vi "Main.vi"(11 "Module Admin":refnum<class "Delacor_lib_QMH_Module Admin.lvclass">) -> ()   [LabVIEW 2021, in "Panther Dashboard.lvlib"]
doc: "Panther Dashboard For DQMH®\n\nDeveloped and maintained by:\nPantherLAB\n\nMain Contributor- Developer:\n\n» Enrique Noé Arias\n\nBrainstorming & Code Reviews:\n\n» Matthias Baudot\n» Fabiola De La Cueva\n» Christopher Farmer\n» Cyril Gambini\n» Joerg Hampel\n» Olivier Jourdan\n» Cesar Muñoz\n» Darren Nattinger\n» Luis Orozco\n» Sam Taggart\n» Diego Torres"
uses:
  Panther Dashboard.lvlib
  <vilib>/Delacor/Delacor QMH/Libraries/Module Admin_class/Delacor_lib_QMH_Module Admin.lvclass
  Window Position--enum.ctl
  Module Data--cluster.ctl
  Maps List and refs--cluster.ctl
  <vilib>/National Instruments/Tree Map/Tree Map Data.ctl
  DQMH Modules Info--cluster.ctl
  Module type--enum.ctl
  Project References--cluster.ctl
  Selection Type--enum.ctl
  References Updated Argument--cluster.ctl
  Launch DQMH Scripting Tools Argument--cluster.ctl
  DQMH Tools Menu--enum.ctl
  <vilib>/Delacor/Delacor QMH/Libraries/Message Queue_class/Delacor_lib_QMH_Message Queue.lvclass/Delacor_lib_QMH_Message Queue.ctl
  Expand Results Argument--cluster.ctl
  Execute Default Event Request Argument--cluster.ctl
  Tree DQMH Selection Argument--cluster.ctl
  Scan DQMH Modules Argument--cluster.ctl
  Stop Argument--cluster.ctl
  Generate Project Documentation Argument--cluster.ctl
  Set App Theme Argument--cluster.ctl
  Show About Argument--cluster.ctl
  Update Module ID Argument--cluster.ctl
  Save Library Description Argument--cluster.ctl
  Save VI Description Argument--cluster.ctl
  Open Documentation Argument--cluster.ctl
  Save Project Documentation Argument--cluster.ctl
  Update Window Position Argument--cluster.ctl
  Public VIs names--enum.ctl
  <vilib>/Delacor/Delacor QMH/Libraries/Module Admin_class/Delacor_lib_QMH_Module Admin.lvclass/Delacor_lib_QMH_Module Admin.ctl
  <vilib>/Delacor/Delacor QMH/Libraries/Message Queue_class/Delacor_lib_QMH_Enqueue Message (Single).vi
  <vilib>/Delacor/Delacor QMH/Libraries/Module Admin_class/Delacor_lib_QMH_Get External Launch.vi
  Panther Dashboard--global.vi
  <vilib>/Platform/browser.llb/Open URL in Default Browser (path).vi
  <vilib>/Utility/error.llb/Error Cluster From Error Code.vi
  <vilib>/ErrorRing/Error Ring.xnode
  <vilib>/Delacor/Delacor QMH/Libraries/Message Queue_class/Delacor_lib_QMH_Message Queue.lvclass
  <vilib>/National Instruments/Tree Map/Tree Map.lvlib
  <vilib>/Delacor/Delacor QMH/Libraries/Scripting API/DQMH_Scripting API.lvlib
  ContextHelp/ContextHelp.lvlib
panel:
  out "error out":errorcluster
  in  "Context Help Panther":bool caption="Doc Editor"
  in  "Add Event":bool
  in  "Remove Event":bool caption="Remove"
  in  "Convert Event":bool caption="Convert"
  in  "Rename Event":bool caption="Rename"
  in  "Add Helper Loop to Module":bool
  in  "Add New Module":bool caption="Add"
  in  "Rename Module":bool caption="Rename"
  in  "Validate Module":bool caption="Validate"
  in  "Create Module Template":bool caption="Template"
  in  "Add Unit Test Module":bool caption="Unit Test"
  in  "Create RT Tester Module":bool caption="RT Tester"
  in  "Open Antidoc Output":bool caption="Open"
  in  "Generate Antidoc":bool caption="Antidoc"
  in  "About Panther":bool caption="About"
  in  "Theme Panther":bool caption="Theme"
  in  "Projects":string(combo)
  in  "Targets":string(combo)
  in  "Expand Results":bool
  in  "Include Dependencies":bool
  in  "Search All":bool caption="Scan All in Project"
  in  "Search":bool caption="Manual Scan Project"
  in  "Module ID":i32=-1 min=-1 max=1000 step=1 format="Module ID %d"
  in  "Modules Tree":string(tree) caption="Tree 2"
  out "antidoc":bool
  out "Panther Indicator":bool
  out "Process Indicator":bool
  out "Event Indicator":bool
  out "Status":string
  out "Progress":u16(slide) scale=-1.0..3.0
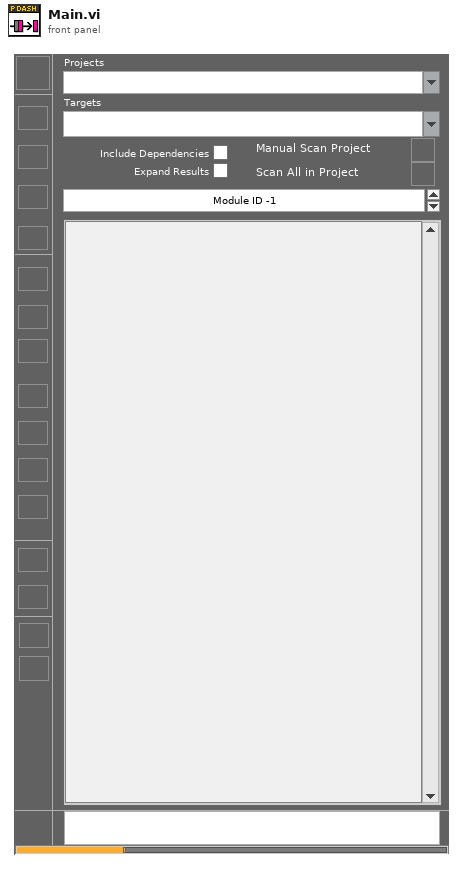
[diagram p1: front panel]
types:
  T1 = typedef "Panther Dashboard.lvlib/Window Position--enum.ctl" = enum16{"Right", "Left", "Max"}
  T2 = typedef "Panther Dashboard.lvlib/Broadcast Events--cluster.ctl" = cluster{"Module Did Init":refnum<user-event>, "Status Updated":refnum<user-event>, "Error Reported":refnum<user-event>, "Module Did Stop":refnum<user-event>, "Update Module Execution Status":refnum<user-event>, "References Updated":refnum<user-event>, "Projects Updated":refnum<user-event>, "Targets Updated":refnum<user-event>, "Progress updated":refnum<user-event>, "Scale Updated":refnum<user-event>, "Connector Pane Updated":refnum<user-event>, "Documentation Updated":refnum<user-event>, "Module Type Updated":refnum<user-event>, "Theme Updated":refnum<user-event>, "Project Description Updated":refnum<user-event>}
  T3 = typedef "Panther Dashboard.lvlib/Request Events--cluster.ctl" = cluster{"Stop Module":refnum<user-event>, "Show Panel":refnum<user-event>, "Hide Panel":refnum<user-event>, "Get Module Execution Status":refnum<user-event>, "Show Diagram":refnum<user-event>, "Scan DQMH Modules":refnum<user-event>, "Tree DQMH Selection":refnum<user-event>, "Open Module API Tester":refnum<user-event>, "Execute Default Event Request":refnum<user-event>, "Expand Results":refnum<user-event>, "Launch DQMH Scripting Tools":refnum<user-event>, "Generate Project Documentation":refnum<user-event>, "Set App Theme":refnum<user-event>, "Show About":refnum<user-event>, "Update Module ID":refnum<user-event>, "Save Library Description":refnum<user-event>, "Save VI Description":refnum<user-event>, "Open Documentation":refnum<user-event>, "Save Project Documentation":refnum<user-event>, "Register controls Mouse Enter":refnum<user-event>, "Update Window Position":refnum<user-event>}
  T4 = typedef "ContextHelp.lvlib/Broadcast Events--cluster.ctl" = cluster{"Module Did Init":refnum<user-event>, "Status Updated":refnum<user-event>, "Error Reported":refnum<user-event>, "Module Did Stop":refnum<user-event>, "Update Module Execution Status":refnum<user-event>}
  T5 = typedef "Panther Dashboard.lvlib/Selection Type--enum.ctl" = enum16{"Broadcast", "Request", "Module", "Public API"}
  T6 = typedef "Panther Dashboard.lvlib/Module Data--cluster.ctl" = cluster{"Maps":T7, "DQMH Scan Results":T9, "Current Selection":cluster{"VI Ref":refnum<vi>, "DQMH Lib Ref":refnum<vi>}, "Module type":T10, "Module ID":i32, "Theme":bool, "Broadcast?":bool}
  T7 = typedef "Panther Dashboard.lvlib/Maps List and refs--cluster.ctl" = cluster{"Tree Map":T8, "References Map":map{string, refnum<vi>}}
  T8 = typedef "Tree Map.lvlib/Tree Map Data.ctl" = map{string, cluster{"Child Paths Set":set{string}, "Name":string, "Data":string, "Attributes":map{string, string}}}
  T9 = typedef "Panther Dashboard.lvlib/DQMH Modules Info--cluster.ctl" = cluster{"All DQMH Modules Refs":refnum<vi>[], "All Modules Descriptions":string[], "All Modules type":T10[], "Project References":T11, "Dependencies":bool[]}
  T10 = typedef "Panther Dashboard.lvlib/Module type--enum.ctl" = enum16{"Module type: Singleton", "Module type: Cloneable"}
  T11 = typedef "Panther Dashboard.lvlib/Project References--cluster.ctl" = cluster{"Project Ref":refnum<vi>, "Project Name":string, "Target":refnum<vi>, "App Ref":refnum<vi>}
  T12 = typedef "Panther Dashboard.lvlib/References Updated Argument--cluster.ctl" = cluster{"Modules":refnum<vi>[], "Modules Types":T10[], "Application Instance":refnum<vi>, "Dependencies":bool[]}
  T13 = enum8{"Enabled", "Disabled", "Disabled and Grayed Out"}
  T14 = typedef "Panther Dashboard.lvlib/Launch DQMH Scripting Tools Argument--cluster.ctl" = cluster{"Scripting Tool":T15}
  T15 = typedef "Panther Dashboard.lvlib/DQMH Tools Menu--enum.ctl" = enum16{"Create New DQMH Event", "Remove DQMH Event", "Convert DQMH Event", "Rename DQMH Event", "Add New DQMH Module", "Create RT Tester", "Rename DQMH Module", "Validate DQMH Module", "Create DQMH Module Template", "New DQMH  Unit Test", "Add Helper Loop to DQMH Module"}
  T16 = typedef "Panther Dashboard.lvlib/Expand Results Argument--cluster.ctl" = cluster{"Expand?":bool}
  T17 = typedef "Panther Dashboard.lvlib/Execute Default Event Request Argument--cluster.ctl" = cluster{"Event Name":string}
  T18 = typedef "Panther Dashboard.lvlib/Tree DQMH Selection Argument--cluster.ctl" = cluster{"Tree DQMH Sel":string}
  T19 = typedef "Panther Dashboard.lvlib/Scan DQMH Modules Argument--cluster.ctl" = cluster{"Include Dependencies":bool, "Project":string, "Target":string, "All":bool}
  T20 = enum32{"invalid lock state", "Not Locked", "Locked (No Password)", "Password-protected"}
  T21 = typedef "Panther Dashboard.lvlib/Stop Argument--cluster.ctl" = cluster{"Origin":string, "Exit via Stop Module Req?":bool, "Wait for Module to stop?":bool}
  T22 = typedef "Panther Dashboard.lvlib/Generate Project Documentation Argument--cluster.ctl" = cluster{"Boolean":bool}
  T23 = typedef "Panther Dashboard.lvlib/Set App Theme Argument--cluster.ctl" = cluster{"Theme":bool}
  T24 = typedef "Panther Dashboard.lvlib/Show About Argument--cluster.ctl" = cluster{"Boolean":bool}
  T25 = typedef "Panther Dashboard.lvlib/Update Module ID Argument--cluster.ctl" = cluster{"New ID":i32}
  T26 = typedef "Panther Dashboard.lvlib/Save Library Description Argument--cluster.ctl" = cluster{"Library Description":string}
  T27 = typedef "Panther Dashboard.lvlib/Save VI Description Argument--cluster.ctl" = cluster{"VI Description":string}
  T28 = typedef "Panther Dashboard.lvlib/Open Documentation Argument--cluster.ctl" = cluster{"Boolean":bool}
  T29 = typedef "Panther Dashboard.lvlib/Save Project Documentation Argument--cluster.ctl" = cluster{"Project Description":string}
  T30 = typedef "Panther Dashboard.lvlib/Update Window Position Argument--cluster.ctl" = cluster{"Window Position":T1}
  T31 = typedef "Panther Dashboard.lvlib/Public VIs names--enum.ctl" = enum16{"Start Module.vi", "Synchronize Module Events.vi", "Obtain Broadcast Events for Registration.vi", "Null Broadcast Events--constant.vi", "Stop Module.vi"}
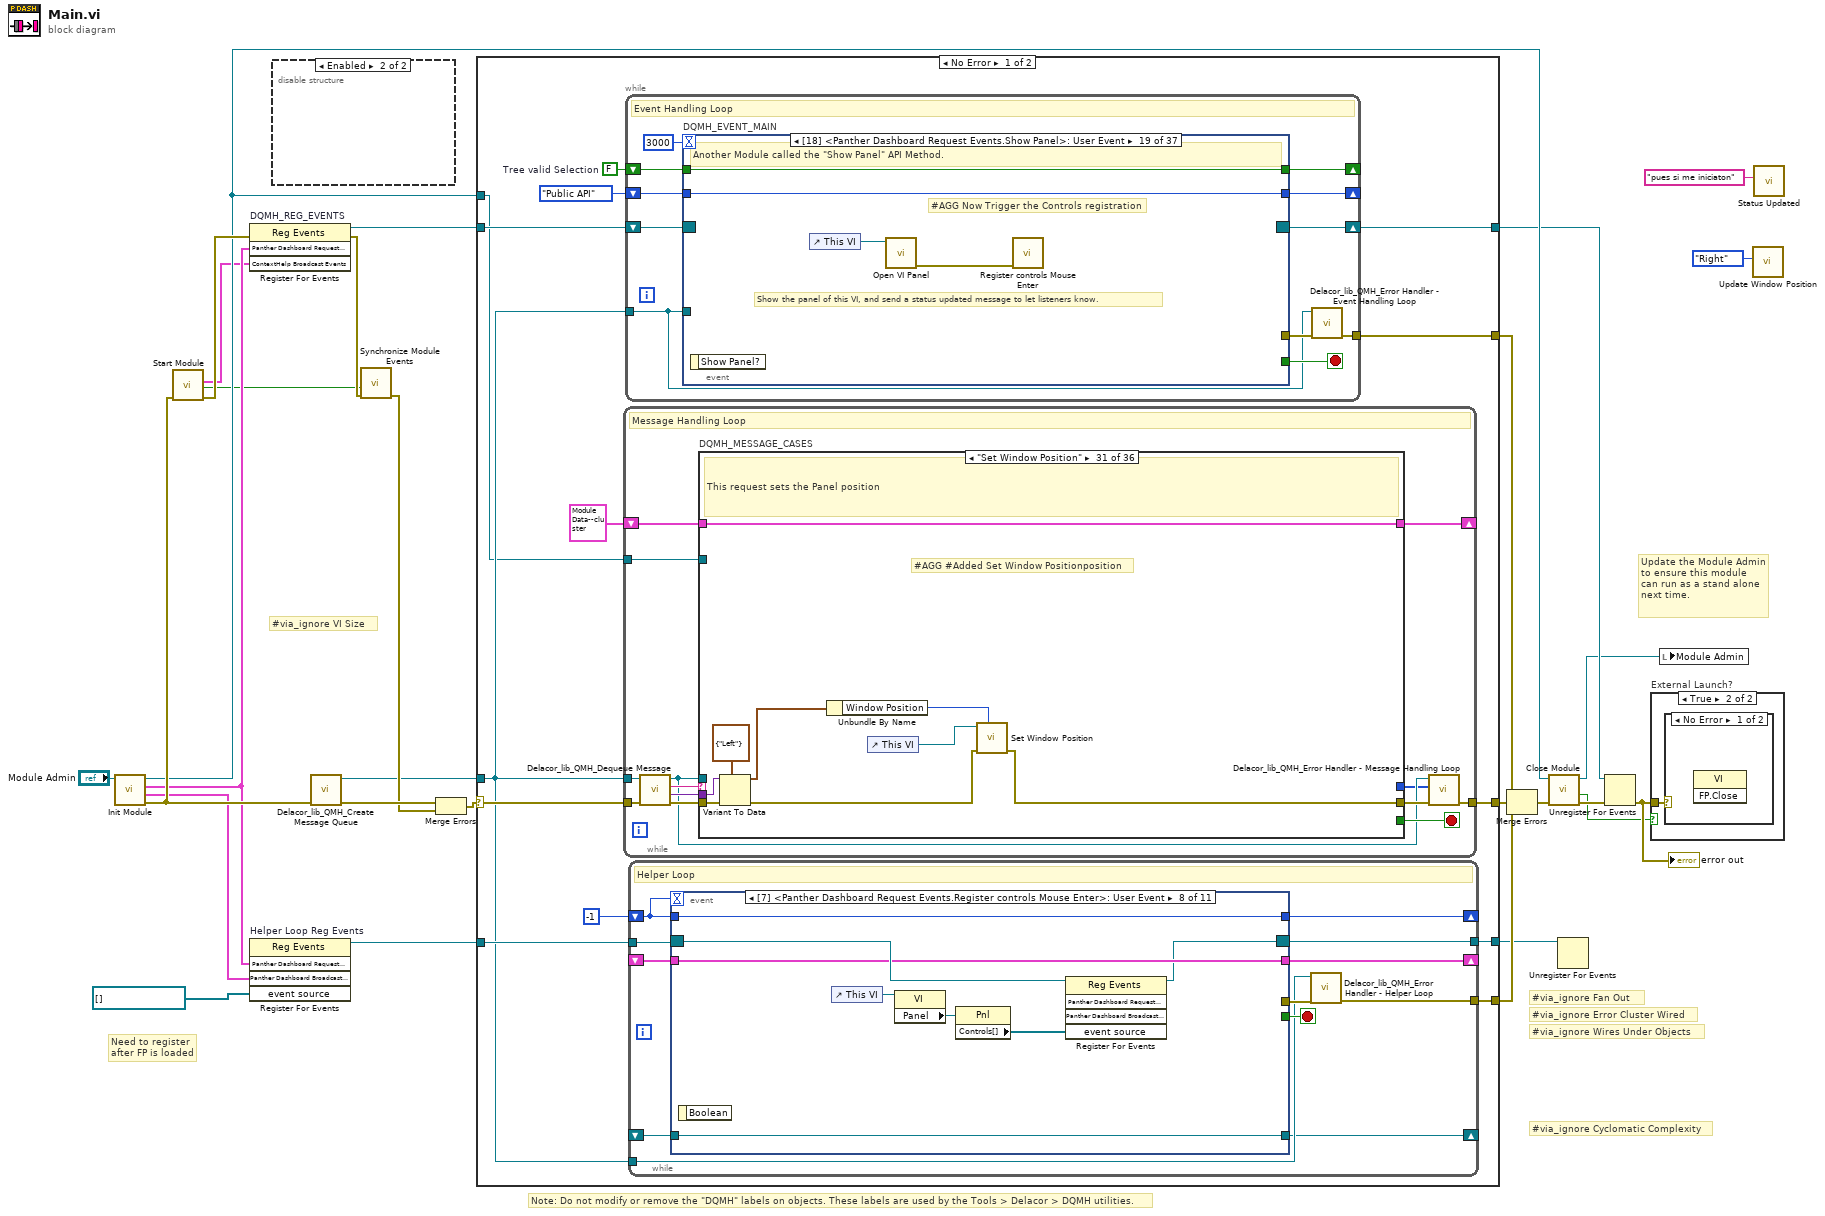
[diagram p0: block diagram]
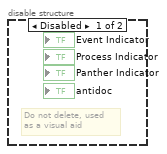
[diagram p2: hidden frame]
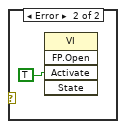
[diagram p4: hidden frame]
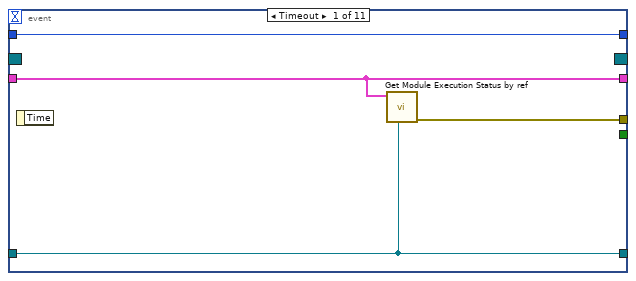
[diagram p5: hidden frame]
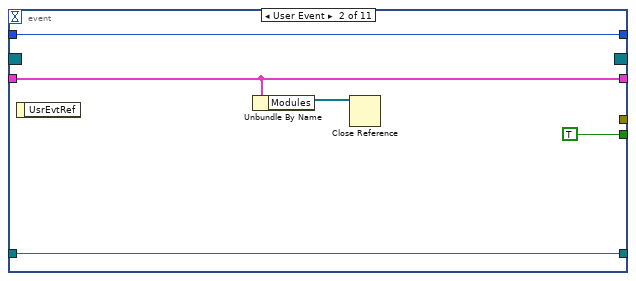
[diagram p6: hidden frame]
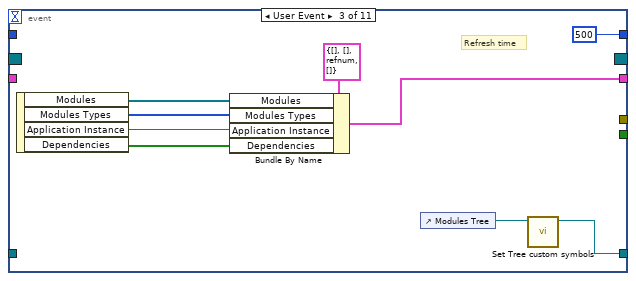
[diagram p7: hidden frame]
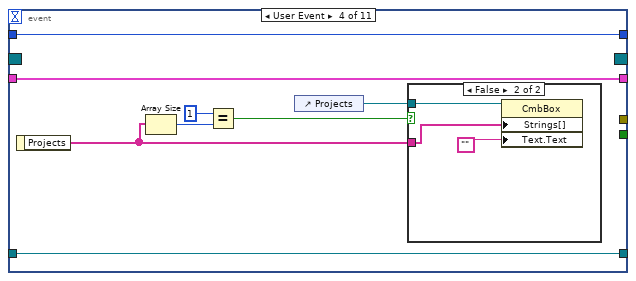
[diagram p8: hidden frame]
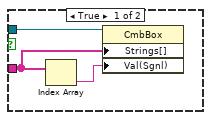
[diagram p9: hidden frame]
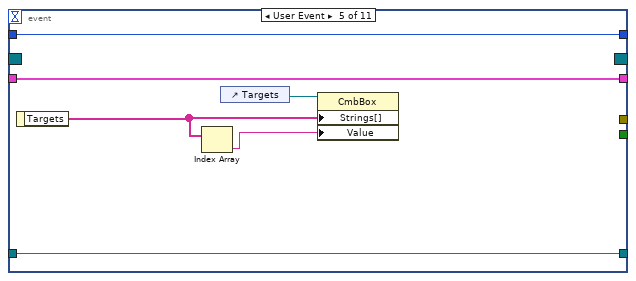
[diagram p10: hidden frame]
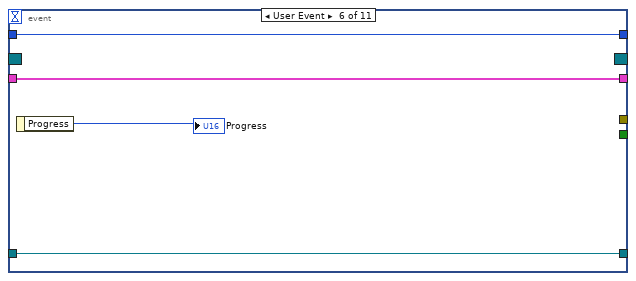
[diagram p11: hidden frame]
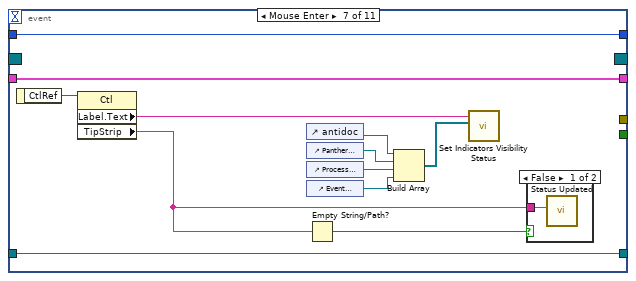
[diagram p12: hidden frame]
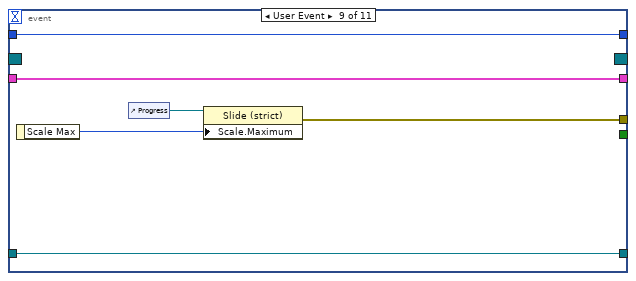
[diagram p14: hidden frame]
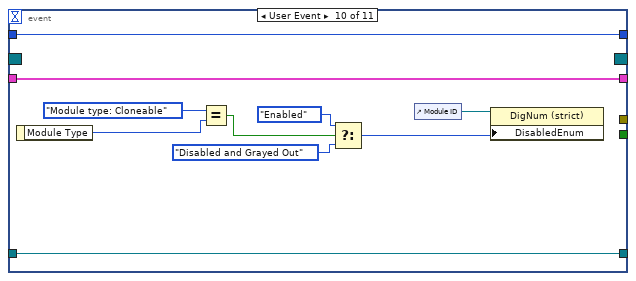
[diagram p15: hidden frame]
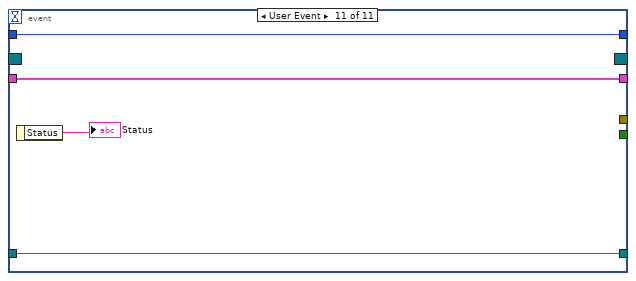
[diagram p16: hidden frame]
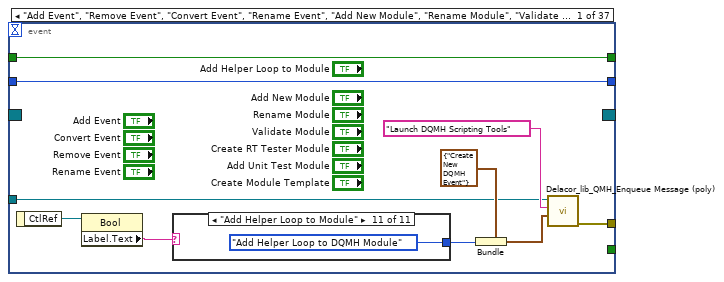
[diagram p17: hidden frame]
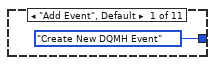
[diagram p18: hidden frame]
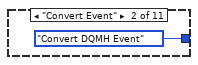
[diagram p19: hidden frame]
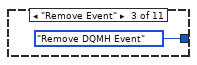
[diagram p20: hidden frame]
diagram:
  # "Need to register\nafter FP is loaded"
  # "#via_ignore VI Size"
  # "#via_ignore Fan Out"
  # "#via_ignore Cyclomatic Complexity"
  # "#via_ignore Wires Under Objects"
  # "#via_ignore Error Cluster Wired"
  # "Note: Do not modify or remove the \"DQMH\" labels on objects. These labels are used by the Tools > Delacor > DQMH utilities."
  # "Update the Module Admin to ensure this module can run as a stand alone next time."
  n1 = call "Init Module.vi"("Singleton Module Admin in"="Module Admin") -> ("error out"=w17:errorcluster, "Panther Dashboard Broadcast Events"=w6:T2, "Panther Dashboard Request Events"=w7:T3, "Singleton Module Admin out"=w16:refnum<class "Delacor_lib_QMH_Module Admin.lvclass">)  [unwired: 7 in]
  n2 = call "Start Module.vi"("error in"=w17) -> ("error out"=w19:errorcluster, "Wait for Event Sync?"=w5:bool, "ContextHelp Broadcast Events"=w4:T4)  [unwired: 7 in, 1 out]
  n3 = register-events "DQMH_REG_EVENTS"(error in=w19, w7, w4) -> (reference out=w14:refnum<event-registration>, error out=w20:errorcluster)  [unwired: 1 in]
  n4 = register-events "Helper Loop Reg Events"(w7, w6, refnum<vi>[] [] ("event source")) -> (reference out=w9:refnum<event-registration>)  [unwired: 2 in, 1 out]
  n5 = disable-structure shown="Enabled" {
    frame Disabled {
      # "Do not delete, used\nas a visual aid"
    }
    frame Enabled {
    }
  }
  n6 = call <vilib>:"Delacor_lib_QMH_Create Message Queue.vi"("error in"=w17) -> ("error out"=w23:errorcluster, "Message Queue"=w13:refnum<class "Delacor_lib_QMH_Message Queue.lvclass">)  [unwired: 9 in]
  n7 = call "Synchronize Module Events.vi"("error in"=w20, "Wait for Event Sync?"=w5) -> ("error out"=w18:errorcluster)  [unwired: 9 in]
  n8 = Merge Errors(w23, w18) -> (w22:errorcluster)
  n9 = case shown="No Error" w22 {
    selector: w22 -> [w40 w852]
    tunnel: [w42 w851] -> w28
    tunnel: [w38 w850] -> w15
    tunnel: w14 -> [w36 w850]
    tunnel: w13 -> [w32 w846]
    tunnel: [w41 _] -> w26
    tunnel: w16 -> [w29 w847]
    tunnel: w9 -> [w35 w845]
    tunnel: [w34 w845] -> w8
    tunnel: [w39 _] -> w21
    frame No Error {
      w31 = FALSE  # Tree valid Selection
      n10 = while {
        tunnel: w32 -> [w461]
        shift-right: [w465] -> _
        shift-left: T6 {"Maps"={"Tree Map"={}, "References Map"={}}, "DQMH Scan Results"={"All DQMH Modules Refs"=[], "All Modules Descriptions"=[], "All Modules type"=[], "Project References"={"Project Ref"=refnum, "Project Name"="", "Target"=refnum, "App Ref"=refnum}, "Dependencies"=[]}, "Current Selection"={"VI Ref"=refnum, "DQMH Lib Ref"=refnum}, "Module type"=enum."Module type: Singleton", "Module ID"=0, "Theme"=FALSE, "Broadcast?"=FALSE} ("Data Cluster") -> [w466]
        tunnel: w40 -> [w469]
        tunnel: [w467] -> w42
        tunnel: w29 -> [w459]
        stop <- w464 stop-if-true
        # "Message Handling Loop"
        n11 = call-dynamic "Delacor_lib_QMH_Dequeue Message.vi"("error in"=w469, "Message Queue in"=w461) -> ("error out"=w468:errorcluster, "Message Data"=w462:variant, "Message"=w463:string, "Message Queue out"=w460:refnum<class "Delacor_lib_QMH_Message Queue.lvclass">)  [unwired: 6 in]
        n12 = case "DQMH_MESSAGE_CASES" shown="\"Set Window Position\"" w463 {
          selector: w463 -> [_ w501 _ _ _ _ _ _ _ _ _ _ _ _ _ _ _ _ _ _ _ _ _ _ _ _ _ _ _ _ _ _ _ _ _ w831]
          tunnel: w460 -> [_ _ _ _ _ _ _ _ _ _ _ _ _ _ _ _ _ _ _ _ _ _ _ _ _ _ _ _ _ _ _ _ _ w800 w823 _]
          tunnel: w468 -> [w495 w506 w508 w521 w533 w540 w547 w554 w561 w576 w585 w590 w596 w610 w623 w645 w651 w657 w665 w672 w677 w690 w699 w710 w722 w730 w740 w756 w772 w783 w792 w795 w797 w807 w829 w833]
          tunnel: [w486 w504 w508 w510 w532 w539 w547 w554 w561 w575 w584 w591 w597 w608 w612 w646 w650 w658 w664 w671 w676 w688 w697 w707 w718 w729 w738 w754 w771 w781 w786 w794 w797 w803 w826 w834] -> w470
          tunnel: w466 -> [w489 w503 w507 w514 w531 w537 w546 w553 w560 w571 w583 w589 w595 w603 w622 w644 w649 w655 w663 w670 w675 w679 w693 w706 w717 w728 w732 w749 w761 w777 w791 w793 w796 w802 w815 w832]
          tunnel: [w493 w503 w507 w513 w530 w537 w546 w553 w560 w567 w583 w589 w595 w603 w622 w644 w649 w655 w661 w670 w675 w679 w693 w701 w717 w724 w731 w747 w761 w777 w791 w793 w796 w802 w815 w832] -> w465
          tunnel: [_ _ _ _ _ _ _ _ _ _ _ _ _ _ _ _ _ _ _ _ _ _ _ _ _ _ _ _ _ _ _ _ _ _ w822 _] -> w464
          tunnel: w462 -> [_ w502 _ w520 _ _ _ _ _ w574 _ _ _ w606 _ _ _ _ w662 w669 _ w687 w695 w705 w716 w727 w736 w752 w770 w780 w790 _ _ w801 w821 _]
          tunnel: w459 -> [w494 _ _ _ _ _ _ _ _ _ _ _ _ _ _ _ _ _ _ _ _ _ _ _ _ _ _ _ _ _ _ _ _ w799 w816 _]
          tunnel: [_ _ _ _ _ _ _ _ _ _ _ _ _ _ i32[] [5000, 1026, 43] ("specific error code to clear (0: all)") _ _ _ _ _ _ _ _ _ _ _ _ _ _ _ _ _ _ _ _ _] -> w458
          frame "Initialize" {
            # "Initialize - Any operation that needs to be done before the module can receive messages. Synchronize Caller Events.vi will inform Start Module.vi that the module has launched and is ready to receive messages. Module Did Init.vi will broadcast that the module initialized."
            n13 = call "Synchronize Caller Events.vi"("error in (no error)"=w495, "Singleton Module Admin in"=w494) -> ("error out"=w485:errorcluster)  [unwired: 8 in, 1 out]
            n14 = property on="Modules Tree" class="Tree (strict)"("Allow Item Drag"=TRUE ("Drag/Drop:Allow Dragging"), "SelColor"=u32 8355711) -> ()  [unwired: 2 in, 2 out]
            n15 = call "Module Name--constant.vi"() -> ("Module Name"=w483:string)  [unwired: 11 in]
            n16 = call "Module Did Init.vi"("error in (no error)"=w485, "Initialized?"=TRUE, "Origin"=w483) -> ("error out"=w482:errorcluster)  [unwired: 8 in]
            n17 = control-ref of="Projects"() -> (w478:refnum<vi>)
            n18 = control-ref of="Add Helper Loop to Module"() -> (w488:refnum<vi>)
            n19 = call "Scan For App Projects.vi"("error in"=w482, "Init?"=TRUE, "Projects Ref"=w478) -> ("error out"=w481:errorcluster)  [unwired: 8 in]
            n20 = call "Read Theme from Config.vi"("error in"=w481) -> ("error out"=w480:errorcluster, "Theme"=w475:bool)  [unwired: 9 in]
            n21 = local write "Theme Panther"(w475) -> ()
            n22 = call "Set App Theme.vi"("error in"=w480, "Theme"=w475) -> ("error out"=w472:errorcluster)  [unwired: 9 in]
            n23 = Build Array(w488) -> (w487:refnum<vi>[])
            n24 = call "Enable DQMH Version Caracteristics.vi"("Ctl Array"=w487) -> ()  [unwired: 11 in]
            n25 = control-ref of="This VI"() -> (w474:refnum<vi>)
            n26 = call "Update Window Position.vi"("error in"=w472, "Window Position"=Window_Position--enum."Right") -> ("error out"=w471:errorcluster)  [unwired: 9 in]
            n27 = flat-sequence {
              tunnel: [w498] -> w479
              tunnel: "Panther Dashboard for DQMH" ("format string") -> [w497]
              tunnel: w474 -> [w496]
              tunnel: w471 -> [_]
              frame #0 {
                n28 = call "Status Updated.vi"("Status"=w497) -> ()  [unwired: 10 in, 1 out]
                n29 = call "Set Panel Initial State.vi"("Title"=w497, "Main Vi Ref"=w496) -> ("error out"=w498:errorcluster)  [unwired: 9 in]
              }
            }
            n30 = Bundle By Name(cluster=w489, "Module ID"=-1) -> (w493:T6)
            n31 = Merge Errors(w479, w471) -> (w486:errorcluster)
          }
          frame "Refresh Targets" {
            # "When the User selects a Project triggers this task to scan all the targets available"
            n32 = Variant To Data(error in=w506, type=w501, Variant=w502) -> (data=w500:string, error out=w505:errorcluster)
            n33 = call "Get all Targets.vi"("error in"=w505, "Project Selection"=w500) -> ("error out"=w504:errorcluster, "Targets"=w499:string[])  [unwired: 8 in]
            n34 = call "Targets Updated.vi"("Targets"=w499) -> ()  [unwired: 10 in, 1 out]
          }
          frame "---Module Specific---" {
            # "Separator -- The following cases handle messages specific to this Module."
          }
          frame "Scan DQMH Modules" {
            # "Scan DQMH Modules in the project and fill 2 maps one with the Vi References and the another one with the list of DQMH modules on the project"
            n35 = Variant To Data(error in=w521, type=T19 {"Include Dependencies"=FALSE, "Project"="", "Target"="", "All"=FALSE} ("Scan DQMH Modules Argument"), Variant=w520) -> (data=w518:T19, error out=w511:errorcluster)
            n36 = Unbundle By Name(w518) -> ("Project"=w515:string, "Target"=w516:string, "Include Dependencies"=w517:bool, "All"=w509:bool)
            n37 = call <vilib>:"Set Busy.vi"("error in (no error)"=w511) -> ()  [unwired: 9 in, 2 out]
            n38 = control-ref of="Modules Tree"() -> (w512:refnum<vi>)
            n39 = call "Scan DQMH Modules and create Maps.vi"("All"=w509, "TreeControl in"=w512, "Data Cluster In"=w514, "error in"=w511, "Include Dependencies"=w517, "Target Selection"=w516, "Project"=w515) -> ("error out"=w510:errorcluster, "Data Cluster Out"=w513:T6)  [unwired: 3 in]
            n40 = call <vilib>:"Unset Busy.vi"("error in (no error)"=w510) -> ()  [unwired: 10 in, 1 out]
            n41 = local write "Include Dependencies"(w517) -> ()
          }
          frame "Refresh Module" {
            # "User right click a module and selected Refresh module"
            n42 = Unbundle By Name(w531) -> ("DQMH Scan Results.Project References.App Ref"=w524:refnum<vi>, "Current Selection.DQMH Lib Ref"=w525:refnum<vi>, "Maps.Tree Map"=w527:T8, "Maps.References Map"=w526:map{string, refnum<vi>})
            n43 = local read "Expand Results"() -> (w523:bool)
            n44 = control-ref of="Modules Tree"() -> (w522:refnum<vi>)
            n45 = call "Refresh Current DQMH Module.vi"("TreeControl in"=w522, "App Ref"=w524, "Expand Results"=w523, "DQMH Lib Ref"=w525, "error in"=w533, "References Map"=w526, "Tree Map In"=w527) -> ("error out"=w532:errorcluster, "map ref out"=w529:map{string, refnum<vi>}, "Tree Map out"=w528:T8)  [unwired: 2 in]
            n46 = Bundle By Name(cluster=w531, "Maps.Tree Map"=w528, "Maps.References Map"=w529) -> (w530:T6)
          }
          frame "Drag VI" {
            # "This is the functionality alowing drag and drop the current selection to your code, you can build code using panther Dashboard."
            n47 = Unbundle By Name(w537) -> ("DQMH Scan Results.Project References.App Ref"=w536:refnum<vi>, "DQMH Scan Results.Project References.Target"=w535:refnum<vi>, "Current Selection.VI Ref"=w534:refnum<vi>)
            n48 = call "Drop Event into subVI.vi"("Current Selection.VI Ref"=w534, "Target"=w535, "App Ref"=w536) -> ("error out"=w538:errorcluster)  [unwired: 8 in]
            n49 = Merge Errors(w538, w540) -> (w539:errorcluster)
          }
          frame "Where is this module being Launched?" {
            # "Find all the VIS calling the Start Module.vi of the selected module library"
            n50 = Unbundle By Name(w546) -> ("Theme"=w545:bool, "DQMH Scan Results.Project References.App Ref"=w544:refnum<vi>, "DQMH Scan Results.Project References.Target"=w543:refnum<vi>, "Current Selection.DQMH Lib Ref"=w542:refnum<vi>)
            n51 = call "Find some Public API VI.vi"("Theme"=w545, "Framework VI to Find"=Public_VIs_names--enum."Start Module.vi", "Library in"=w542, "Target"=w543, "App Ref"=w544) -> ()  [unwired: 7 in]
          }
          frame "Find Code registered to this module's broadcasts" {
            # "Find all the VIS calling the Obtain broadcast events for registration of the selected module library"
            n52 = Unbundle By Name(w553) -> ("Theme"=w551:bool, "DQMH Scan Results.Project References.App Ref"=w550:refnum<vi>, "DQMH Scan Results.Project References.Target"=w549:refnum<vi>, "Current Selection.DQMH Lib Ref"=w548:refnum<vi>)
            n53 = call "Find some Public API VI.vi"("Theme"=w551, "Framework VI to Find"=Public_VIs_names--enum."Obtain Broadcast Events for Registration.vi", "Library in"=w548, "Target"=w549, "App Ref"=w550) -> ()  [unwired: 7 in]
          }
          frame "Where is this module being Stopped?" {
            # "Find all the VIS calling the Obtain broadcast events for registration of the selected module library"
            n54 = Unbundle By Name(w560) -> ("Theme"=w558:bool, "DQMH Scan Results.Project References.App Ref"=w557:refnum<vi>, "DQMH Scan Results.Project References.Target"=w556:refnum<vi>, "Current Selection.DQMH Lib Ref"=w555:refnum<vi>)
            n55 = call "Find some Public API VI.vi"("Theme"=w558, "Framework VI to Find"=Public_VIs_names--enum."Stop Module.vi", "Library in"=w555, "Target"=w556, "App Ref"=w557) -> ()  [unwired: 7 in]
          }
          frame "Tree DQMH Selection" {
            # "There is a new selection of the DQMH Tree list, need to search and update indicators acordanly."
            n56 = Unbundle By Name(w571) -> ("Maps.Tree Map"=w570:T8, "Maps.References Map"=w569:map{string, refnum<vi>}, "DQMH Scan Results"=w568:T9)
            n57 = Variant To Data(error in=w576, type=T18 {"Tree DQMH Sel"=""} ("Tree DQMH Selection Argument"), Variant=w574) -> (data=w572:T18, error out=w575:errorcluster)
            n58 = Unbundle By Name(w572) -> ("Tree DQMH Sel"=w565:string)
            n59 = call "Get List Information.vi"("List Selection"=w565, "DQMH Scan Info"=w568, "References Map"=w569, "Tree Map"=w570) -> ("Broadcast?"=w564:bool, "Vi out"=w563:refnum<vi>, "Module type"=w562:T10, "DQMH Lib"=w566:refnum<vi>)  [unwired: 4 in]
            n60 = Bundle By Name(cluster=w571, "Current Selection.DQMH Lib Ref"=w566, "Module type"=w562, "Current Selection.VI Ref"=w563, "Broadcast?"=w564) -> (w567:T6)
          }
          frame "Open Module API Tester" {
            # "If nothing selected use the first DQMH module"
            # "Open the API Tester from the current DQMH Module Selected"
            n61 = Unbundle By Name(w583) -> ("DQMH Scan Results.Project References.App Ref"=w582:refnum<vi>, "DQMH Scan Results.All DQMH Modules Refs"=w581:refnum<vi>[], "Current Selection.DQMH Lib Ref"=w577:refnum<vi>)
            n62 = Index Array(array=w581) -> (element=w579:refnum<vi>)  [unwired: 1 in]
            n63 = Not A Number/Path/Refnum?(number/path/refnum=w577) -> (NaN/Path/Refnum?=w580:bool)
            n64 = Select(t=w579, s=w580, f=w577) -> (s? t:f=w578:refnum<vi>)
            n65 = call "Open API Tester.vi"("error in"=w585, "DQMH Library Ref"=w578, "Application Instance"=w582) -> ("error out"=w584:errorcluster)  [unwired: 8 in]
          }
          frame "Find Module in project" {
            # "Find the selected module in project explorer"
            n66 = Unbundle By Name(w589) -> ("Current Selection.DQMH Lib Ref"=w588:refnum<vi>, "DQMH Scan Results.Project References.Project Ref"=w587:refnum<vi>, "DQMH Scan Results.All DQMH Modules Refs"=w586:refnum<vi>[])
            n67 = call "Find Library in Project.vi"("error in (no error)"=w590, "DQMH Modules Refs"=w586, "Project Ref"=w587, "DQMH Lib Ref"=w588) -> ("error out"=w591:errorcluster)  [unwired: 7 in]
          }
          frame "Locate Event on Main" {
            # "Find the selected event vi on the owing DQMH Module, if it is a reques we highlight its frame, if it is a broadcast we highlight where the broadcast is being triggered"
            n68 = Unbundle By Name(w595) -> ("DQMH Scan Results.Project References.App Ref"=w593:refnum<vi>, "Current Selection.VI Ref"=w594:refnum<vi>, "Broadcast?"=w592:bool)
            n69 = call "Find Event Frame.vi"("error in"=w596, "Broadcast?"=w592, "VI in"=w594, "Application Instance"=w593) -> ("error out"=w597:errorcluster)  [unwired: 7 in]
          }
          frame "Execute Default Event Request" {
            # "Execute Default Event"
            n70 = Variant To Data(error in=w610, type=T17 {"Event Name"=""} ("Execute Default Event Request Argument"), Variant=w606) -> (data=w604:T17, error out=w609:errorcluster)
            n71 = Unbundle By Name(w603) -> ("DQMH Scan Results.Project References.App Ref"=w602:refnum<vi>, "Current Selection.DQMH Lib Ref"=w601:refnum<vi>, "Module ID"=w599:i32, "Module type"=w598:T10)
            n72 = Unbundle By Name(w604) -> ("Event Name"=w600:string)
            n73 = call "Execute Default event.vi"("Module type"=w598, "Module ID"=w599, "Event"=w600, "DQMH Library Ref"=w601, "application Instance"=w602) -> ("error out"=w607:errorcluster)  [unwired: 6 in]
            n74 = Merge Errors(w609, w607) -> (w608:errorcluster)
          }
          frame "Search for Event Callers / listeners" {
            # "1026-Invalid Ref\n43- Operation\n canceled by user\n5000- something\nrandom happening\non DQMH Scripting\nAPI"
            # "Search for this event callers"
            n75 = Unbundle By Name(w622) -> ("DQMH Scan Results.Project References.Project Ref"=w616:refnum<vi>, "Current Selection.VI Ref"=w621:refnum<vi>, "Theme"=w613:bool, "Broadcast?"=w614:bool)
            n76 = Select(t="Searching code registered to broadcast selection" ("Status"), s=w614, f="Searching for Event Callers" ("Status")) -> (s? t:f=w617:string)
            n77 = call "Status Updated.vi"("error in (no error)"=w623, "Status"=w617) -> ("error out"=w611:errorcluster)  [unwired: 9 in]
            n78 = case shown="True" w614 {
              tunnel: w611 -> [w628 w635]
              tunnel: [w627 w634] -> w612
              tunnel: w621 -> [w626 w631]
              tunnel: [w625 w633] -> w620
              tunnel: w616 -> [w624 w632]
              frame False {
                # "Requests"
                n79 = call <vilib>:"Get Callers of Request VI in Project.vi"("error in"=w628, "Request VI"=w626, "Project"=w624) -> ("error out"=w627:errorcluster, "Request VI Callers"=w625:refnum<vi>[])  [unwired: 7 in]
              }
              frame True {
                # "Broadcast"
                n80 = Two Button Dialog(message="This is an exhaustive task that can take up to minutes, do you wish to continue?") -> (T button?=w630:bool)  [unwired: 2 in]
                n81 = case shown="True" w630 {
                  tunnel: w635 -> [w636 w641]
                  tunnel: [w636 w640] -> w634
                  tunnel: [_ w639] -> w633
                  tunnel: w632 -> [_ w638]
                  tunnel: w631 -> [_ w637]
                  frame False {
                  }
                  frame True {
                    n82 = call <vilib>:"Get VIs Registered for Broadcast in Project.vi"("error in"=w641, "Broadcast VI"=w637, "Project"=w638) -> ("error out"=w640:errorcluster, "VIs Registered for Broadcast"=w639:refnum<vi>[])  [unwired: 7 in]
                  }
                }
              }
            }
            n83 = call <vilib>:"Set Busy.vi"("error in (no error)"=w611) -> ()  [unwired: 9 in, 2 out]
            n84 = call <vilib>:"Unset Busy.vi"("error in (no error)"=w612) -> ()  [unwired: 10 in, 1 out]
            n85 = call "Start Call to results window.vi"("Find Broadcast?"=w614, "Request VI Callers"=w620, "Event"=w621, "Theme"=w613) -> ()  [unwired: 8 in]
          }
          frame "Open VI on Disk" {
            # "Open current event selection on the file system"
            n86 = Unbundle By Name(w644) -> ("Current Selection.VI Ref"=w643:refnum<vi>)
            n87 = property class="VI"(reference=w643) -> ("Path"=w642:path)  [unwired: 1 in, 2 out]
            n88 = call "Open File on Disk.vi"("error in"=w645, "file or directory path"=w642) -> ("error out"=w646:errorcluster)  [unwired: 9 in]
          }
          frame "Open File Library on Disk" {
            # "Open current Module Library selection on the file system"
            n89 = Unbundle By Name(w649) -> ("Current Selection.DQMH Lib Ref"=w648:refnum<vi>)
            n90 = property class="Library"(reference=w648) -> ("Path"=w647:path)  [unwired: 1 in, 2 out]
            n91 = call "Open File on Disk.vi"("error in"=w651, "file or directory path"=w647) -> ("error out"=w650:errorcluster)  [unwired: 9 in]
          }
          frame "Open Event Arguments" {
            # "Open The event selected DQMH Arguments, also open the Event BD to do edits on it"
            n92 = Unbundle By Name(w655) -> ("Current Selection.VI Ref"=w654:refnum<vi>)
            n93 = property on="Property Node" class="VI"(reference=w654, error in=w657, "BDWin.Open"=TRUE ("Block Diagram Window:Open")) -> (reference out=w652:refnum<vi>, error out=w656:errorcluster)
            n94 = call "Open Event Arguments.vi"("error in (no error)"=w656, "VI Refnum"=w652) -> ("error out"=w658:errorcluster)  [unwired: 9 in]
          }
          frame "Module ID Update" {
            # "Module ID Control has value change"
            n95 = Variant To Data(error in=w665, type=0 ("Module ID"), Variant=w662) -> (data=w660:i32, error out=w664:errorcluster)
            n96 = Bundle By Name(cluster=w663, "Module ID"=w660) -> (w661:T6)
          }
          frame "Expand or Close" {
            # "Expand or Close DQMH Tree control"
            n97 = Variant To Data(error in=w672, type=T16 {"Expand?"=FALSE} ("Expand or Close Argument"), Variant=w669) -> (data=w667:T16, error out=w671:errorcluster)
            n98 = Unbundle By Name(w667) -> ("Expand?"=w666:bool)
            n99 = invoke on="Modules Tree" class="Tree (strict)" method="Open/Close.Open/Close All"("Open"=w666) -> ()  [unwired: 3 in, 4 out]
          }
          frame "Open Project Folder" {
            n100 = Unbundle By Name(w675) -> ("DQMH Scan Results.Project References.Project Ref"=w674:refnum<vi>)
            n101 = property class="Project"(reference=w674) -> ("Path"=w673:path)  [unwired: 1 in, 2 out]
            n102 = call "Open File on Disk.vi"("error in"=w677, "file or directory path"=w673) -> ("error out"=w676:errorcluster)  [unwired: 9 in]
          }
          frame "Launch DQMH Scripting Tools" {
            # "Launch the DQMH Scripting Tools"
            n103 = Variant To Data(error in=w690, type=T14 {"Scripting Tool"=enum."Create New DQMH Event"} ("Launch DQMH Scripting Tools Argument"), Variant=w687) -> (data=w685:T14, error out=w689:errorcluster)
            n104 = Unbundle By Name(w685) -> ("Scripting Tool"=w680:T15)
            n105 = Unbundle By Name(w679) -> ("DQMH Scan Results.Project References.Project Name"=w683:string, "DQMH Scan Results.Project References.App Ref"=w684:refnum<vi>, "Current Selection.DQMH Lib Ref"=w678:refnum<vi>)
            n106 = Format Into String(format string="DQMH Tool: %s being executed ", w680) -> (resulting string=w682:string)  [unwired: 2 in, 1 out]
            n107 = call "Status Updated.vi"("Status"=w682) -> ()  [unwired: 10 in, 1 out]
            n108 = call "Launch DQMH Tools by menu.vi"("Project"=w683, "Application Instance"=w684, "error in"=w689, "Module Ref"=w678, "DQMH Tools"=w680) -> ("error out"=w688:errorcluster)  [unwired: 6 in]
          }
          frame "Generate Project Documentation" {
            n109 = Variant To Data(error in=w699, type=T22 {"Boolean"=FALSE} ("Generate Project Documentation Argument"), Variant=w695) -> (error out=w698:errorcluster)  [unwired: 1 out]
            n110 = Unbundle By Name(w693) -> ("DQMH Scan Results.Project References.Project Ref"=w692:refnum<vi>)
            n111 = property class="Project"(reference=w692) -> ("Path"=w691:path)  [unwired: 1 in, 2 out]
            n112 = call "Generate Documentation--dialog.vi"("Project Path"=w691) -> ("error out"=w696:errorcluster)  [unwired: 10 in]
            n113 = Merge Errors(w698, w696) -> (w697:errorcluster)
          }
          frame "Set App Theme" {
            # "#AGG the FP might be closed"
            # "Set Panther Dashboard Theme"
            n114 = Variant To Data(error in=w710, type=T23 {"Theme"=FALSE} ("Set App Theme Argument"), Variant=w705) -> (data=w703:T23, error out=w708:errorcluster)
            n115 = Unbundle By Name(w703) -> ("Theme"=w700:bool)
            n116 = control-ref of="This VI"() -> (w702:refnum<vi>)
            n117 = Bundle By Name(cluster=w706, "Theme"=w700) -> (w701:T6)
            n118 = call "Set Theme.vi"("Dark?"=w700, "VI in"=w702) -> ()  [unwired: 10 in]
            n119 = call "Theme Updated.vi"("Theme"=w700) -> ()  [unwired: 10 in, 1 out]
            n120 = call "Save Theme in config.vi"("error in"=w708, "Theme"=w700) -> ("error out"=w709:errorcluster)  [unwired: 9 in]
            n121 = disable-structure shown="Disabled" {
              disable-tunnel: w709 -> [w712 w713]
              disable-tunnel: [w711 w713] -> w707
              frame Disabled {
                n122 = call "Register controls Mouse Enter.vi"("error in"=w712) -> ("error out"=w711:errorcluster)  [unwired: 10 in]
              }
              frame Enabled {
              }
            }
          }
          frame "Show About" {
            # "Show About project"
            n123 = Variant To Data(error in=w722, type=T24 {"Boolean"=FALSE} ("Show About Argument"), Variant=w716) -> (error out=w719:errorcluster)  [unwired: 1 out]
            n124 = control-ref of="This VI"() -> (w714:refnum<vi>)
            n125 = call "Hide VI Panel.vi"("error in (no error)"=w719, "VI"=w714) -> ("error out"=w721:errorcluster)  [unwired: 9 in]
            n126 = call "About Panther Dashboard.vi"("error in"=w721) -> ("error out"=w720:errorcluster)  [unwired: 10 in]
            n127 = call "Open VI Panel.vi"("error in (no error)"=w720, "VI"=w714) -> ("error out"=w718:errorcluster)  [unwired: 9 in]
          }
          frame "Update Module ID" {
            # "Update the Current Module ID"
            n128 = Variant To Data(error in=w730, type=T25 {"New ID"=-1} ("Update Module ID Argument"), Variant=w727) -> (data=w725:T25, error out=w729:errorcluster)
            n129 = Unbundle By Name(w725) -> ("New ID"=w723:i32)
            n130 = Bundle By Name(cluster=w728, "Module ID"=w723) -> (w724:T6)
          }
          frame "Save Library Description" {
            # "Save Library Description"
            n131 = Variant To Data(error in=w740, type=T26 {"Library Description"=""} ("Save Library Description Argument"), Variant=w736) -> (data=w734:T26, error out=w739:errorcluster)
            n132 = Unbundle By Name(w734) -> ("Library Description"=w733:string)
            n133 = in-place {
              in-place-border: w733 -> [w744]
              in-place-border: [w746] -> w737
              n134 = in-place-cluster #1(w732) -> ("Current Selection.DQMH Lib Ref"=w745:refnum<vi>, "DQMH Scan Results"=w742:T9)
              n135 = call "Save Library Documentation.vi"("New Description"=w744, "DQMH Modules Info In"=w742, "Library in"=w745) -> ("error out"=w746:errorcluster, "DQMH Modules Info Out"=w743:T9, "Lib out"=w741:refnum<vi>)  [unwired: 6 in]
              n136 = in-place-cluster #1("Current Selection.DQMH Lib Ref"=w741, "DQMH Scan Results"=w743) -> (w731:T6)
            }
            n137 = Merge Errors(w739, w737) -> (w738:errorcluster)
          }
          frame "Save VI Description" {
            # "Save Event Description"
            n138 = Variant To Data(error in=w756, type=T27 {"VI Description"=""} ("Save VI Description Argument"), Variant=w752) -> (data=w750:T27, error out=w755:errorcluster)
            n139 = Unbundle By Name(w750) -> ("VI Description"=w748:string)
            n140 = in-place {
              in-place-border: w748 -> [w759]
              in-place-border: [w760] -> w753
              n141 = in-place-cluster #2(w749) -> ("Current Selection.VI Ref"=w758:refnum<vi>)
              n142 = call "Save Event Description.vi"("Event Description"=w759, "Event Ref in"=w758) -> ("error out"=w760:errorcluster, "Event Ref out"=w757:refnum<vi>)  [unwired: 8 in]
              n143 = in-place-cluster #2("Current Selection.VI Ref"=w757) -> (w747:T6)
            }
            n144 = Merge Errors(w755, w753) -> (w754:errorcluster)
          }
          frame "Open Documentation" {
            # "Open Antidoc Documentation"
            n145 = Variant To Data(error in=w772, type=T28 {"Boolean"=FALSE} ("Open Documentation Argument"), Variant=w770) -> (error out=w771:errorcluster)  [unwired: 1 out]
            n146 = Unbundle By Name(w761) -> ("DQMH Scan Results.Project References.Project Ref"=w768:refnum<vi>)
            n147 = property class="Project"(reference=w768) -> ("Path"=w767:path)  [unwired: 1 in, 2 out]
            n148 = Strip Path(path=w767) -> (stripped path=w766:path)  [unwired: 1 out]
            n149 = Build Path(base path=w766, name or relative path=path "Antidoc-Output/Project-Documentation.pdf") -> (appended path=w765:path)
            n150 = call <vilib>:"Check if File or Folder Exists.vi"("path"=w765) -> ("file or folder exists?"=w763:bool, "dup path"=w764:path)  [unwired: 8 in, 1 out]
            n151 = case shown="False" w763 {
              tunnel: w764 -> [_ w774]
              frame False {
                n152 = invoke on="Generate Antidoc" class="Bool" method="ObjHighlight"() -> ()  [unwired: 3 in, 3 out]
                n153 = call "Status Updated.vi"("Status"="No Antidoc Output has been found, please select a project and generate it first.") -> ()  [unwired: 10 in, 1 out]
              }
              frame True {
                n154 = call-poly <vilib>:"Open URL in Default Browser.vi"("path"=w774) -> ()  [unwired: 5 in, 2 out]
              }
            }
          }
          frame "Save Project Documentation" {
            n155 = Variant To Data(error in=w783, type=T29 {"Project Description"=""} ("Save Project Documentation Argument"), Variant=w780) -> (data=w778:T29, error out=w782:errorcluster)
            n156 = Unbundle By Name(w778) -> ("Project Description"=w775:string)
            n157 = Unbundle By Name(w777) -> ("DQMH Scan Results.Project References.Project Ref"=w776:refnum<vi>)
            n158 = property class="Project"(reference=w776, error in=w782, "Description"=w775) -> (error out=w781:errorcluster)  [unwired: 1 out]
          }
          frame "Set Window Position" {
            # "#AGG #Added Set Window Positionposition"
            # "This request sets the Panel position"
            n159 = Variant To Data(error in=w792, type=T30 {"Window Position"=enum."Left"} ("Set Window Position Argument"), Variant=w790) -> (data=w788:T30, error out=w787:errorcluster)
            n160 = Unbundle By Name(w788) -> ("Window Position"=w784:T1)
            n161 = control-ref of="This VI"() -> (w785:refnum<vi>)
            n162 = call "Set Window Position.vi"("Module type"=w784, "error in (no error)"=w787, "Vi reference"=w785) -> ("error out"=w786:errorcluster)  [unwired: 8 in]
          }
          frame "---Copy This Frame---" {
            # "Duplicate this frame when creating new messages.  Change this comment in the duplicated frame to describe this message."
            n163 = Merge Errors(w795) -> (w794:errorcluster)
          }
          frame "---Exit and Error Handling---" {
            # "Separator - The following cases handle errors and exit messages."
          }
          frame "Error" {
            # "Error - Check the error message data and respond accordingly. This message is sent by the \"Error Handler\" VIs at the end of each loop in this application."
            n164 = property on="Property Node" class="Module Admin"(reference=w799) -> ("Accessors:External Launch"=w798:bool)  [unwired: 1 in, 2 out]
            n165 = Variant To Data(error in=w807, type=errorcluster {"status"=FALSE, "code"=0, "source"=""} ("error constant"), Variant=w801) -> (data=w808:errorcluster, error out=w805:errorcluster)
            n166 = call "Error Reported.vi"("Error"=w808) -> ()  [unwired: 10 in, 1 out]
            n167 = case shown="True" w798 {
              tunnel: [w813 _] -> w804
              tunnel: w800 -> [w811 _]
              tunnel: w808 -> [w812 _]
              frame False {
                # "If the module is running standalone, then pop up an error dialog and call the \"Exit\" message."
                n168 = call <vilib>:"Simple Error Handler.vi"("error in (no error)"=w812) -> ()  [unwired: 4 in, 5 out]
                n169 = call-poly <vilib>:"Delacor_lib_QMH_Enqueue Message (poly).vi"("Priority Message? (F)"=TRUE, "Message"="Exit", "Message Queue in"=w811) -> ("error out"=w813:errorcluster)  [unwired: 7 in, 1 out]
              }
              frame True {
                # "If the module was launched externally, calling the Error Reported broadcast VI is the only action performed by the \"Error\" message. The module's caller can then process the error appropriately."
              }
            }
            n170 = Merge Errors(w805, w804) -> (w803:errorcluster)
            n171 = local write "error out"(w803) -> ()
          }
          frame "Exit" {
            w820 = 91  # 91: not all Exit messages will have an argument
            w822 = TRUE  # Stop the VI
            # "Release the message queue reference"
            # "Exit - Exit the application."
            n172 = Variant To Data(error in=w829, type=T21 {"Origin"="", "Exit via Stop Module Req?"=FALSE, "Wait for Module to stop?"=FALSE} ("Stop Argument"), Variant=w821) -> (data=w818:T21, error out=w825:errorcluster)
            n173 = call <vilib>:"Clear Errors.vi"("error in (no error)"=w825, "specific error code to clear (0: all)"=w820) -> ("error out"=w828:errorcluster)  [unwired: 4 in, 1 out]
            n174 = control-ref of="This VI"() -> (w817:refnum<vi>)
            n175 = invoke on="Modules Tree" class="Tree (strict)" method="Edit Tree Items.Delete"() -> ()  [unwired: 5 in, 5 out]
            n176 = call-dynamic "Delacor_lib_QMH_Release Message Queue.vi"("error in"=w828, "Message Queue"=w823) -> ("error out"=w827:errorcluster)  [unwired: 9 in]
            n177 = call "Handle Exit.vi"("Stop Argument"=w818, "Admin in"=w816, "VI reference"=w817) -> ("error out"=w824:errorcluster)  [unwired: 7 in, 1 out]
            n178 = call "Close vi references.vi"("Data Cluster"=w815) -> ()  [unwired: 10 in, 1 out]
            n179 = Merge Errors(w827, w824) -> (w826:errorcluster)
            n180 = call "Stop Module.vi"("Origin"="Panther Dahsboard Stopped") -> ()  [unwired: 10 in, 1 out]
          }
          frame Default {
            # "'Default' case only runs if there is a message that isn't defined in any of the other cases.  Output a programming error."
            n181 = call "Module Name--constant.vi"() -> ("Module Name"=w830:string)  [unwired: 11 in]
            n182 = xnode ("Error Ring")("parameter 0"=w831, "parameter 1"=w830) -> ("error out"=w835:errorcluster)
            n183 = Merge Errors(w833, w835) -> (w834:errorcluster)
          }
        }
        n184 = call-dynamic "Delacor_lib_QMH_Error Handler - Message Handling Loop.vi"("error in"=w470, "Ignore Errors (Runtime)"=w458, "Message Queue in"=w460) -> ("dup error in"=w467:errorcluster)  [unwired: 7 in, 1 out]
      }
      n185 = while {
        tunnel: w32 -> [w143]
        shift-right: [w145] -> w38
        shift-left: w36 -> [w146]
        tunnel: [w147] -> w41
        shift-right: [w141] -> _
        shift-left: w31 -> [w140]
        shift-right: [w139] -> _
        shift-left: Selection_Type--enum."Public API" ("Selection type") -> [w138]
        stop <- w144 stop-if-true
        # "Event Handling Loop"
        n186 = event "DQMH_EVENT_MAIN" shown="[18] <Panther Dashboard Request Events.Show Panel>: User Event" {
          selector: w146 -> [_ _ _ _ _ _ _ _ _ _ _ _ _ _ _ _ _ _ _ _ _ _ _ _ _ _ _ _ _ _ _ _ _ _ _ _ _]
          dyn-events: [_ _ _ _ _ _ _ _ _ _ _ _ _ _ _ _ _ _ _ _ _ _ _ _ _ _ _ _ _ _ _ _ _ _ _ _ _] -> w145
          timeout: 3000 -> [_ _ _ _ _ _ _ _ _ _ _ _ _ _ _ _ _ _ _ _ _ _ _ _ _ _ _ _ _ _ _ _ _ _ _ _ _]
          tunnel: [_ _ _ _ _ _ _ _ _ _ _ _ _ _ _ _ _ _ _ TRUE ("Discard?") _ _ _ _ _ _ _ _ _ _ _ _ _ _ _ _ _] -> w144
          tunnel: w143 -> [w149 _ _ w185 w190 w202 w207 w226 _ w235 _ w249 w259 _ _ w277 w287 _ _ w322 w331 _ w342 w350 w358 w366 w374 w382 w390 w398 w406 w414 w422 w430 w438 w446 w455]
          tunnel: [w158 w173 w178 w186 w191 w203 w208 w227 w232 w238 w246 w252 w260 w264 _ w278 w288 _ _ w325 w333 w337 w345 w353 w361 w369 w377 w385 w393 w401 w409 w417 w425 w433 w441 w449 w450] -> w148
          tunnel: [w157 w172 w177 w180 w188 w199 w205 w222 w228 w237 w245 w251 w254 w262 w266 w271 w285 w301 w313 w315 w328 w336 w344 w352 w360 w368 w376 w384 w392 w400 w408 w416 w424 w432 w440 w448 w457] -> w141
          tunnel: w140 -> [w157 w172 w177 w180 w188 w199 w205 _ w228 w237 w245 w251 w254 w262 w266 w271 w285 w301 w313 w315 w328 w336 w344 w352 w360 w368 w376 w384 w392 w400 w408 w416 w424 w432 w440 w448 w457]
          tunnel: [w156 w171 w176 w179 w187 w198 w204 w220 w230 w236 w244 w250 w253 w261 w265 w270 w284 w300 w312 w314 w327 w335 w343 w351 w359 w367 w375 w383 w391 w399 w407 w415 w423 w431 w439 w447 w456] -> w139
          tunnel: w138 -> [w156 w171 w176 w179 _ w198 w204 _ w230 w236 w244 w250 w253 w261 w265 w270 w284 w300 w312 w314 w327 w335 w343 w351 w359 w367 w375 w383 w391 w399 w407 w415 w423 w431 w439 w447 w456]
          event "Add Event", "Remove Event", "Convert Event", "Rename Event", "Add New Module", "Rename Module", "Validate Module", "Create Module Template", "Add Unit Test Module", "Create RT Tester Module", "Add Helper Loop to Module": Value Change {
            n187 = event-data() -> ("CtlRef"=w154:refnum<vi>)  [unwired: 1 in]
            n188 = property class="Bool"(reference=w154) -> ("Label.Text"=w155:string)  [unwired: 1 in, 2 out]
            n189 = case shown="\"Add Helper Loop to Module\"" w155 {
              tunnel: [DQMH_Tools_Menu--enum."Create New DQMH Event" ("DQMH Tools") DQMH_Tools_Menu--enum."Convert DQMH Event" ("DQMH Tools") DQMH_Tools_Menu--enum."Remove DQMH Event" ("DQMH Tools") DQMH_Tools_Menu--enum."Rename DQMH Event" ("DQMH Tools") DQMH_Tools_Menu--enum."Add New DQMH Module" ("DQMH Tools") DQMH_Tools_Menu--enum."Rename DQMH Module" ("DQMH Tools") DQMH_Tools_Menu--enum."Validate DQMH Module" ("DQMH Tools") DQMH_Tools_Menu--enum."Create RT Tester" ("DQMH Tools") DQMH_Tools_Menu--enum."New DQMH  Unit Test" ("DQMH Tools") DQMH_Tools_Menu--enum."Create DQMH Module Template" ("DQMH Tools") DQMH_Tools_Menu--enum."Add Helper Loop to DQMH Module" ("DQMH Tools")] -> w150
              frame "Add Event", Default {
              }
              frame "Convert Event" {
              }
              frame "Remove Event" {
              }
              frame "Rename Event" {
              }
              frame "Add New Module" {
              }
              frame "Rename Module" {
              }
              frame "Validate Module" {
              }
              frame "Create RT Tester Module" {
              }
              frame "Add Unit Test Module" {
              }
              frame "Create Module Template" {
              }
              frame "Add Helper Loop to Module" {
              }
            }
            n190 = Bundle(cluster=T14 {"Scripting Tool"=enum."Create New DQMH Event"} ("Launch DQMH Scripting Tools Argument"), "Scripting Tool"=w150) -> (w153:T14)
            n191 = call-poly <vilib>:"Delacor_lib_QMH_Enqueue Message (poly).vi"("Message Data"=w153, "Message"="Launch DQMH Scripting Tools", "Message Queue in"=w149) -> ("error out"=w158:errorcluster)  [unwired: 7 in, 1 out]
          }
          event "Context Help Panther": Value Change {
            # "Open Documentation DQMH Module"
            n192 = event-data() -> ()  [unwired: 1 in, 1 out]
            n193 = case shown="True" "Context Help Panther" {
              tunnel: [w174 w175] -> w173
              frame False {
                n194 = call "Hide Panel.vi"() -> ("error out"=w174:errorcluster)  [unwired: 11 in]
              }
              frame True {
                n195 = call "Show Panel.vi"() -> ("error out"=w175:errorcluster)  [unwired: 11 in]
              }
            }
          }
          event User Event {
            # "We wait for the Context help module to init to request to refresh \npanther Dashboard Broadcasts, we need this module to be\nlistening Panther Dashboard broadcasts"
            n196 = event-data() -> ()  [unwired: 1 in, 1 out]
            n197 = call "Refresh Panther Dashboard Broadcasts.vi"() -> ("error out"=w178:errorcluster)  [unwired: 11 in]
          }
          event "Expand Results": Value Change {
            # "Expand or close Result tree"
            n198 = event-data() -> ()  [unwired: 1 in, 1 out]
            n199 = Bundle(cluster=T16 {"Expand?"=FALSE} ("Expand or Close Argument"), "Expand?"="Expand Results") -> (w182:T16)
            n200 = call-poly <vilib>:"Delacor_lib_QMH_Enqueue Message (poly).vi"("Message Data"=w182, "Message"="Expand or Close", "Message Queue in"=w185) -> ("error out"=w186:errorcluster)  [unwired: 7 in, 1 out]
          }
          event "Modules Tree": Double Click {
            # "User double click an element on the tree control, we check if it is an event to find its frame on the corresponding DQMH module, we also check if it is a broadcast to find where is being triggered"
            n201 = event-data() -> ("Tag"=w189:string)  [unwired: 1 in]
            n202 = call "Validate if event is selected.vi"("Tree Selection"=w189) -> ("Selection type"=w187:T5)  [unwired: 10 in]
            n203 = case shown="\"Broadcast\", \"Request\"" w187 {
              tunnel: [w194 _ w197] -> w191
              tunnel: w190 -> [w193 _ w196]
              frame "Module" {
                # "Selection is a module"
                n204 = call-poly <vilib>:"Delacor_lib_QMH_Enqueue Message (poly).vi"("Message"="Find Module in project", "Message Queue in"=w193) -> ("error out"=w194:errorcluster)  [unwired: 8 in, 1 out]
              }
              frame "Public API" {
              }
              frame "Broadcast", "Request" {
                # "Selection is an Event vi?"
                n205 = call-poly <vilib>:"Delacor_lib_QMH_Enqueue Message (poly).vi"("Message"="Locate Event on Main", "Message Queue in"=w196) -> ("error out"=w197:errorcluster)  [unwired: 8 in, 1 out]
              }
            }
          }
          event "Modules Tree": Drag Starting? {
            # "Drag current selection to user destination"
            n206 = event-data() -> ()  [unwired: 1 in, 1 out]
            n207 = call-poly <vilib>:"Delacor_lib_QMH_Enqueue Message (poly).vi"("Message"="Drag VI", "Message Queue in"=w202) -> ("error out"=w203:errorcluster)  [unwired: 8 in, 1 out]
            n208 = event-data("Discard?"=TRUE) -> ()  [unwired: 1 in, 1 out]
          }
          event "Modules Tree": Shortcut Menu Selection (User) {
            # "User selects something from the Right Click Shortcut Menu"
            n209 = event-data() -> ("ItemTag"=w206:string)  [unwired: 1 in]
            n210 = case shown="\"-Run: Hide Panel\", \"-Run: Show Diagram\", \"-Run: Show Panel\", \"-Run: Stop Module\"" w206 {
              selector: w206 -> [w211 w217]
              tunnel: w207 -> [w215 w218]
              tunnel: [w216 w219] -> w208
              frame "-Run: Hide Panel", "-Run: Show Diagram", "-Run: Show Panel", "-Run: Stop Module" {
                n211 = Match Pattern(string=w211, regular expression="-Run: ") -> (after substring=w210:string)  [unwired: 1 in, 3 out]
                n212 = Bundle(cluster=T17 {"Event Name"=""} ("Execute Default Event Request Argument"), "Event Name"=w210) -> (w213:T17)
                n213 = call-poly <vilib>:"Delacor_lib_QMH_Enqueue Message (poly).vi"("Message Data"=w213, "Message"="Execute Default Event Request", "Message Queue in"=w215) -> ("error out"=w216:errorcluster)  [unwired: 7 in, 1 out]
              }
              frame Default {
                n214 = call-poly <vilib>:"Delacor_lib_QMH_Enqueue Message (poly).vi"("Message"=w217, "Message Queue in"=w218) -> ("error out"=w219:errorcluster)  [unwired: 8 in, 1 out]
              }
            }
          }
          event "Modules Tree": Value Change {
            w222 = TRUE  # Tree valid Selection
            # "The user selected an item on the tree control"
            n215 = event-data() -> ()  [unwired: 1 in, 1 out]
            n216 = Bundle(cluster=T18 {"Tree DQMH Sel"=""} ("Tree DQMH Selection Argument"), "Tree DQMH Sel"="Modules Tree") -> (w223:T18)
            n217 = call "Validate if event is selected.vi"("Tree Selection"="Modules Tree") -> ("Selection type"=w220:T5)  [unwired: 10 in]
            n218 = call-poly <vilib>:"Delacor_lib_QMH_Enqueue Message (poly).vi"("Message Data"=w223, "Message"="Tree DQMH Selection", "Message Queue in"=w226) -> ("error out"=w227:errorcluster)  [unwired: 7 in, 1 out]
          }
          event "Modules Tree": Shortcut Menu Activation? {
            # "This is wher the shorcut menu is filled, only after the user select a module"
            n219 = event-data() -> ("MenuRef"=w231:refnum<k9>)  [unwired: 1 in]
            n220 = call "Create Tree Shortcut Menu.vi"("Selection type"=w230, "Menu in"=w231) -> ("error out"=w232:errorcluster)  [unwired: 9 in]
            n221 = Not(x=w228) -> (.not. x?=w229:bool)
            n222 = event-data("Discard?"=w229) -> ()  [unwired: 1 in, 1 out]
          }
          event "Projects": Value Change {
            n223 = event-data() -> ()  [unwired: 1 in, 1 out]
            n224 = call-poly <vilib>:"Delacor_lib_QMH_Enqueue Message (poly).vi"("Message Data"="Projects", "Message"="Refresh Targets", "Message Queue in"=w235) -> ("error out"=w238:errorcluster)  [unwired: 7 in, 1 out]
          }
          event "Projects": Shortcut Menu Activation? {
            n225 = event-data() -> ("MenuRef"=w243:refnum<k9>)  [unwired: 1 in]
            n226 = Delete Menu Items(9:w243) -> (0:w247:errorcluster, 3:w242:refnum<k9>)  [unwired: 3 in]
            n227 = Insert Menu Items(6:w247, 8:string[] ["Open Project Folder"] ("item names"), 9:w242) -> (0:w246:errorcluster)  [unwired: 3 in, 2 out]
            n228 = local read "Projects"() -> (w240:string)
            n229 = Empty String/Path?(string/path=w240) -> (empty?=w239:bool)
            n230 = event-data("Discard?"=w239) -> ()  [unwired: 1 in, 1 out]
          }
          event "Projects": Shortcut Menu Selection (User) {
            n231 = event-data() -> ("ItemTag"=w248:string)  [unwired: 1 in]
            n232 = call-poly <vilib>:"Delacor_lib_QMH_Enqueue Message (poly).vi"("Message"=w248, "Message Queue in"=w249) -> ("error out"=w252:errorcluster)  [unwired: 8 in, 1 out]
          }
          event User Event {
            # "Another Module called the \"Expand or Close\" API Method."
            n233 = event-data() -> ("Expand?"=w255:bool)  [unwired: 1 in]
            n234 = Bundle(cluster=T16 {"Expand?"=FALSE} ("Expand or Close Argument"), "Expand?"=w255) -> (w256:T16)
            n235 = call-poly <vilib>:"Delacor_lib_QMH_Enqueue Message (poly).vi"("Message Data"=w256, "Message"="Expand or Close", "Message Queue in"=w259) -> ("error out"=w260:errorcluster)  [unwired: 7 in, 1 out]
          }
          event User Event {
            # "Another Module called the \"Get Module Execution Status\" API Method."
            n236 = event-data() -> ()  [unwired: 1 in, 1 out]
            n237 = call "Update Module Execution Status.vi"("Running?"=TRUE) -> ("error out"=w264:errorcluster)  [unwired: 10 in]
          }
          event User Event {
            # "Hide the panel of this VI, and send a status updated message to let listeners know."
            # "Another Module called the \"Hide Panel\" API Method."
            n238 = event-data() -> ()  [unwired: 1 in, 1 out]
            n239 = control-ref of="This VI"() -> (w267:refnum<vi>)
            n240 = call "Hide VI Panel.vi"("VI"=w267) -> ()  [unwired: 10 in, 1 out]
          }
          event User Event {
            # "Another Module called the \"Scan DQMH Modules\" API Method."
            n241 = event-data() -> ("Include Dependencies"=w273:bool, "Project"=w272:string, "Target"=w269:string, "All"=w268:bool)  [unwired: 1 in]
            n242 = Bundle(cluster=T19 {"Include Dependencies"=FALSE, "Project"="", "Target"="", "All"=FALSE} ("Scan DQMH Modules Argument"), "Include Dependencies"=w273, "Project"=w272, "Target"=w269, "All"=w268) -> (w274:T19)
            n243 = call-poly <vilib>:"Delacor_lib_QMH_Enqueue Message (poly).vi"("Message Data"=w274, "Message"="Scan DQMH Modules", "Message Queue in"=w277) -> ("error out"=w278:errorcluster)  [unwired: 7 in, 1 out]
          }
          event "Search", "Search All": Value Change {
            # "#via_ignore Unwired Event Nodes"
            # "Another Module called the \"Scan DQMH Modules\" API Method."
            n244 = event-data() -> ()  [unwired: 1 in, 1 out]
            n245 = local read "Projects"() -> (w283:string)
            n246 = Empty String/Path?(string/path="Targets") -> (empty?=w281:bool)
            n247 = global write "Panther Dashboard--global.vi" "Target"("Targets") -> ()
            n248 = Empty String/Path?(string/path=w283) -> (empty?=w286:bool)
            n249 = Or(x=w286, y=w281) -> (x .or. y?=w282:bool)
            n250 = case shown="False" w282 {
              tunnel: [w297 _] -> w288
              tunnel: w287 -> [w296 _]
              tunnel: w283 -> [w291 _]
              tunnel: "Targets" -> [w290 _]
              tunnel: "Search All" -> [w289 _]
              frame False {
                n251 = Bundle(cluster=T19 {"Include Dependencies"=FALSE, "Project"="", "Target"="", "All"=FALSE} ("Scan DQMH Modules Argument"), "Include Dependencies"="Include Dependencies", "Project"=w291, "Target"=w290, "All"=w289) -> (w293:T19)
                n252 = call-poly <vilib>:"Delacor_lib_QMH_Enqueue Message (poly).vi"("Message Data"=w293, "Message"="Scan DQMH Modules", "Message Queue in"=w296) -> ("error out"=w297:errorcluster)  [unwired: 7 in, 1 out]
              }
              frame True {
                n253 = invoke on="Projects" class="CmbBox" method="ObjHighlight"() -> (error out=w299:errorcluster)  [unwired: 3 in, 2 out]
                n254 = invoke on="Targets" class="CmbBox" method="ObjHighlight"(error in=w299) -> ()  [unwired: 2 in, 3 out]
                n255 = call "Status Updated.vi"("Status"="Scanning requires a project and an target please make the selection.\n") -> ()  [unwired: 10 in, 1 out]
              }
            }
          }
          event User Event {
            # "Another Module called the \"Show Diagram\" API Method. This event is used for debugging."
            n256 = event-data() -> ()  [unwired: 1 in, 1 out]
            n257 = disable-structure shown="RUN_TIME_ENGINE==False" {
              frame condition #0 (active) {
                # "functionality not available in exe"
                n258 = invoke on="Invoke Node" class="VI" method="Lock State.Get"() -> (error out=w307:errorcluster, "Get Lock State"=w306:T20, "pwd in cache"=w303:bool)  [unwired: 4 in, 1 out]
                n259 = Equal?(x=T20."Password-protected", y=w306) -> (x = y?=w304:bool)
                n260 = Compound Arithmetic op=AND(w304, invert w303) -> (w302:bool)
                n261 = case shown="False" w302 {
                  tunnel: w307 -> [w309 _]
                  frame False {
                    n262 = property on="Property Node" class="VI"(error in=w309, "BDWin.Open"=TRUE ("Block Diagram Window:Open")) -> ()  [unwired: 1 in, 2 out]
                  }
                  frame True {
                    # "Password-protected VI, and the password is not in the cache. Do not show the diagram."
                  }
                }
              }
              frame condition #1 {
              }
            }
          }
          event User Event {
            # "#AGG Now Trigger the Controls registration"
            # "Show the panel of this VI, and send a status updated message to let listeners know."
            # "Another Module called the \"Show Panel\" API Method."
            n263 = event-data() -> ()  [unwired: 1 in, 1 out]
            n264 = control-ref of="This VI"() -> (w311:refnum<vi>)
            n265 = call "Open VI Panel.vi"("VI"=w311) -> ("error out"=w310:errorcluster)  [unwired: 10 in]
            n266 = call "Register controls Mouse Enter.vi"("error in"=w310) -> ()  [unwired: 10 in, 1 out]
          }
          event User Event {
            # "The Stop Module Event can get fired from the Exit message in the MHL. The queue gets destroyed in that case. If the queue no longer exists, the Enqueue Exit as a priority message will return error 1. It is safe to ignore, because the module is already exiting."
            # "Another Module called the \"Stop Module\" API Method  or the Message Handling Loop below."
            n267 = event-data() -> ("Exit via Stop Module Req?"=w318:bool, "Wait for Module to stop?"=w317:bool)  [unwired: 1 in]
            n268 = Bundle By Name(cluster=T21 {"Origin"="", "Exit via Stop Module Req?"=FALSE, "Wait for Module to stop?"=FALSE} ("Stop Argument"), "Exit via Stop Module Req?"=w318, "Wait for Module to stop?"=w317) -> (w316:T21)
            n269 = call-poly <vilib>:"Delacor_lib_QMH_Enqueue Message (poly).vi"("Priority Message? (F)"=TRUE, "Message Data"=w316, "Message"="Exit", "Message Queue in"=w322) -> ("error out"=w326:errorcluster)  [unwired: 6 in, 1 out]
            n270 = call <vilib>:"Clear Errors.vi"("error in (no error)"=w326, "specific error code to clear (0: all)"=1) -> ("error out"=w325:errorcluster)  [unwired: 4 in, 1 out]
          }
          event Panel Close? {
            w332 = TRUE  # Discard the event, the MHL is responsible for closing and stopping this VI.
            # "Hide the panel or send the 'Exit' message if the user clicks the 'X' on the module main VI panel."
            n271 = event-data() -> ()  [unwired: 1 in, 1 out]
            n272 = call-poly <vilib>:"Delacor_lib_QMH_Enqueue Message (poly).vi"("Priority Message? (F)"=TRUE, "Message"="Exit", "Message Queue in"=w331) -> ("error out"=w333:errorcluster)  [unwired: 7 in, 1 out]
            n273 = event-data ("Event Filter Node")("Discard?"=w332) -> ()  [unwired: 1 in, 1 out]
          }
          event Timeout {
            w334 = FALSE  # Init?
            n274 = event-data() -> ()  [unwired: 1 in, 1 out]
            n275 = call "Scan For App Projects.vi"("Init?"=w334) -> ("error out"=w337:errorcluster)  [unwired: 10 in]
          }
          event User Event {
            # "Another Module called the \"Launch DQMH Scripting Tools\" API Method."
            n276 = event-data() -> ("Scripting Tool"=w338:T15)  [unwired: 1 in]
            n277 = Bundle(cluster=T14 {"Scripting Tool"=enum."Create New DQMH Event"} ("Launch DQMH Scripting Tools Argument"), "Scripting Tool"=w338) -> (w339:T14)
            n278 = call-poly <vilib>:"Delacor_lib_QMH_Enqueue Message (poly).vi"("Message Data"=w339, "Message"="Launch DQMH Scripting Tools", "Message Queue in"=w342) -> ("error out"=w345:errorcluster)  [unwired: 7 in, 1 out]
          }
          event User Event {
            # "Another Module called the \"Generate Project Documentation\" API Method."
            n279 = event-data() -> ("Boolean"=w346:bool)  [unwired: 1 in]
            n280 = Bundle(cluster=T22 {"Boolean"=FALSE} ("Generate Project Documentation Argument"), "Boolean"=w346) -> (w347:T22)
            n281 = call-poly <vilib>:"Delacor_lib_QMH_Enqueue Message (poly).vi"("Message Data"=w347, "Message"="Generate Project Documentation", "Message Queue in"=w350) -> ("error out"=w353:errorcluster)  [unwired: 7 in, 1 out]
          }
          event "Generate Antidoc": Value Change {
            # "Another Module called the \"Generate Project Documentation\" API Method."
            n282 = event-data() -> ()  [unwired: 1 in, 1 out]
            n283 = Bundle(cluster=T22 {"Boolean"=FALSE} ("Generate Project Documentation Argument"), "Boolean"="Generate Antidoc") -> (w355:T22)
            n284 = call-poly <vilib>:"Delacor_lib_QMH_Enqueue Message (poly).vi"("Message Data"=w355, "Message"="Generate Project Documentation", "Message Queue in"=w358) -> ("error out"=w361:errorcluster)  [unwired: 7 in, 1 out]
          }
          event User Event {
            # "Another Module called the \"Set App Theme\" API Method."
            n285 = event-data() -> ("Theme"=w362:bool)  [unwired: 1 in]
            n286 = Bundle(cluster=T23 {"Theme"=FALSE} ("Set App Theme Argument"), "Theme"=w362) -> (w363:T23)
            n287 = call-poly <vilib>:"Delacor_lib_QMH_Enqueue Message (poly).vi"("Message Data"=w363, "Message"="Set App Theme", "Message Queue in"=w366) -> ("error out"=w369:errorcluster)  [unwired: 7 in, 1 out]
          }
          event "Theme Panther": Value Change {
            # "Another Module called the \"Set App Theme\" API Method."
            n288 = event-data() -> ()  [unwired: 1 in, 1 out]
            n289 = Bundle(cluster=T23 {"Theme"=FALSE} ("Set App Theme Argument"), "Theme"="Theme Panther") -> (w371:T23)
            n290 = call-poly <vilib>:"Delacor_lib_QMH_Enqueue Message (poly).vi"("Message Data"=w371, "Message"="Set App Theme", "Message Queue in"=w374) -> ("error out"=w377:errorcluster)  [unwired: 7 in, 1 out]
          }
          event User Event {
            # "Another Module called the \"Show About\" API Method."
            n291 = event-data() -> ("Boolean"=w378:bool)  [unwired: 1 in]
            n292 = Bundle(cluster=T24 {"Boolean"=FALSE} ("Show About Argument"), "Boolean"=w378) -> (w379:T24)
            n293 = call-poly <vilib>:"Delacor_lib_QMH_Enqueue Message (poly).vi"("Message Data"=w379, "Message"="Show About", "Message Queue in"=w382) -> ("error out"=w385:errorcluster)  [unwired: 7 in, 1 out]
          }
          event "About Panther": Value Change {
            # "Another Module called the \"Show About\" API Method."
            n294 = event-data() -> ()  [unwired: 1 in, 1 out]
            n295 = Bundle(cluster=T24 {"Boolean"=FALSE} ("Show About Argument"), "Boolean"="About Panther") -> (w387:T24)
            n296 = call-poly <vilib>:"Delacor_lib_QMH_Enqueue Message (poly).vi"("Message Data"=w387, "Message"="Show About", "Message Queue in"=w390) -> ("error out"=w393:errorcluster)  [unwired: 7 in, 1 out]
          }
          event User Event {
            # "Another Module called the \"Update Module ID\" API Method."
            n297 = event-data() -> ("New ID"=w394:i32)  [unwired: 1 in]
            n298 = Bundle(cluster=T25 {"New ID"=-1} ("Update Module ID Argument"), "New ID"=w394) -> (w395:T25)
            n299 = call-poly <vilib>:"Delacor_lib_QMH_Enqueue Message (poly).vi"("Message Data"=w395, "Message"="Update Module ID", "Message Queue in"=w398) -> ("error out"=w401:errorcluster)  [unwired: 7 in, 1 out]
          }
          event "Module ID": Value Change {
            # "Another Module called the \"Update Module ID\" API Method."
            n300 = event-data() -> ()  [unwired: 1 in, 1 out]
            n301 = Bundle(cluster=T25 {"New ID"=-1} ("Update Module ID Argument"), "New ID"="Module ID") -> (w403:T25)
            n302 = call-poly <vilib>:"Delacor_lib_QMH_Enqueue Message (poly).vi"("Message Data"=w403, "Message"="Update Module ID", "Message Queue in"=w406) -> ("error out"=w409:errorcluster)  [unwired: 7 in, 1 out]
          }
          event User Event {
            # "Another Module called the \"Save Library Description\" API Method."
            n303 = event-data() -> ("Library Description"=w410:string)  [unwired: 1 in]
            n304 = Bundle(cluster=T26 {"Library Description"=""} ("Save Library Description Argument"), "Library Description"=w410) -> (w411:T26)
            n305 = call-poly <vilib>:"Delacor_lib_QMH_Enqueue Message (poly).vi"("Message Data"=w411, "Message"="Save Library Description", "Message Queue in"=w414) -> ("error out"=w417:errorcluster)  [unwired: 7 in, 1 out]
          }
          event User Event {
            # "Another Module called the \"Save VI Description\" API Method."
            n306 = event-data() -> ("VI Description"=w418:string)  [unwired: 1 in]
            n307 = Bundle(cluster=T27 {"VI Description"=""} ("Save VI Description Argument"), "VI Description"=w418) -> (w419:T27)
            n308 = call-poly <vilib>:"Delacor_lib_QMH_Enqueue Message (poly).vi"("Message Data"=w419, "Message"="Save VI Description", "Message Queue in"=w422) -> ("error out"=w425:errorcluster)  [unwired: 7 in, 1 out]
          }
          event User Event {
            # "Another Module called the \"Open Documentation\" API Method."
            n309 = event-data() -> ("Boolean"=w426:bool)  [unwired: 1 in]
            n310 = Bundle(cluster=T28 {"Boolean"=FALSE} ("Open Documentation Argument"), "Boolean"=w426) -> (w427:T28)
            n311 = call-poly <vilib>:"Delacor_lib_QMH_Enqueue Message (poly).vi"("Message Data"=w427, "Message"="Open Documentation", "Message Queue in"=w430) -> ("error out"=w433:errorcluster)  [unwired: 7 in, 1 out]
          }
          event "Open Antidoc Output": Value Change {
            # "Another Module called the \"Open Documentation\" API Method."
            n312 = event-data() -> ()  [unwired: 1 in, 1 out]
            n313 = Bundle(cluster=T28 {"Boolean"=FALSE} ("Open Documentation Argument"), "Boolean"="Open Antidoc Output") -> (w435:T28)
            n314 = call-poly <vilib>:"Delacor_lib_QMH_Enqueue Message (poly).vi"("Message Data"=w435, "Message"="Open Documentation", "Message Queue in"=w438) -> ("error out"=w441:errorcluster)  [unwired: 7 in, 1 out]
          }
          event User Event {
            # "Another Module called the \"Save Project Documentation\" API Method."
            n315 = event-data() -> ("Project Description"=w442:string)  [unwired: 1 in]
            n316 = Bundle(cluster=T29 {"Project Description"=""} ("Save Project Documentation Argument"), "Project Description"=w442) -> (w443:T29)
            n317 = call-poly <vilib>:"Delacor_lib_QMH_Enqueue Message (poly).vi"("Message Data"=w443, "Message"="Save Project Documentation", "Message Queue in"=w446) -> ("error out"=w449:errorcluster)  [unwired: 7 in, 1 out]
          }
          event User Event {
            # "Another Module called the \"Set Window Position\" API Method."
            n318 = event-data() -> ("Window Position"=w451:T1)  [unwired: 1 in]
            n319 = Bundle(cluster=T30 {"Window Position"=enum."Left"} ("Set Window Position Argument"), "Window Position"=w451) -> (w452:T30)
            n320 = call-poly <vilib>:"Delacor_lib_QMH_Enqueue Message (poly).vi"("Message Data"=w452, "Message"="Set Window Position", "Message Queue in"=w455) -> ("error out"=w450:errorcluster)  [unwired: 7 in, 1 out]
          }
        }
        n321 = call-dynamic "Delacor_lib_QMH_Error Handler - Event Handling Loop.vi"("error in"=w148, "Message Queue in"=w143) -> ("dup error in"=w147:errorcluster)  [unwired: 8 in, 1 out]
      }
      n322 = while {
        tunnel: w35 -> [w52]
        tunnel: [w51] -> w34
        shift-right: [w49] -> _
        shift-left: -1 -> [w48]
        shift-right: [w47] -> _
        shift-left: _ -> [w46]
        tunnel: w32 -> [w45]
        tunnel: [w53] -> w39
        shift-right: [w44] -> _
        shift-left: _ -> [w43]
        stop <- w50 stop-if-true
        # "Helper Loop"
        n323 = event shown="[7] <Panther Dashboard Request Events.Register controls Mouse Enter>: User Event" {
          selector: w52 -> [_ _ _ _ _ _ _ w115 _ _ _]
          dyn-events: [_ _ _ _ _ _ _ w113 _ _ _] -> w51
          timeout: w48 -> [_ _ _ _ _ _ _ _ _ _ _]
          tunnel: [_ TRUE _ _ _ _ _ _ _ _ _] -> w50
          tunnel: [w56 w61 w67 w80 w92 w96 w108 w114 w122 w133 w137] -> w47
          tunnel: [w57 w62 500 w79 w91 w95 w107 w117 w121 w132 w136] -> w49
          tunnel: w48 -> [w57 w62 _ w79 w91 w95 w107 w117 w121 w132 w136]
          tunnel: w46 -> [w56 w61 _ w80 w92 w96 w108 w114 w122 w133 w137]
          tunnel: [w58 _ _ _ _ _ _ _ w123 _ _] -> w54
          tunnel: [w55 w59 w65 w78 w89 w94 w106 w116 w120 w131 w135] -> w44
          tunnel: w43 -> [w55 w59 _ w78 w89 w94 w106 w116 w120 w131 w135]
          event Timeout {
            n324 = event-data() -> ()  [unwired: 1 in, 1 out]
            n325 = call "Get Module Execution Status by ref.vi"("Modules Tree ref"=w55, "Refs"=w56) -> ("error out"=w58:errorcluster)  [unwired: 9 in]
          }
          event User Event {
            n326 = event-data() -> ()  [unwired: 1 in, 1 out]
            n327 = Unbundle By Name(w61) -> ("Modules"=w60:refnum<vi>[])
            n328 = Close Reference(reference=w60) -> ()  [unwired: 1 in, 1 out]
          }
          event User Event {
            # "Refresh time"
            n329 = event-data() -> ("Modules"=w70:refnum<vi>[], "Modules Types"=w68:T10[], "Application Instance"=w69:refnum<vi>, "Dependencies"=w64:bool[])  [unwired: 1 in]
            n330 = Bundle By Name(cluster=T12 {"Modules"=[], "Modules Types"=[], "Application Instance"=refnum, "Dependencies"=[]}, "Modules"=w70, "Modules Types"=w68, "Application Instance"=w69, "Dependencies"=w64) -> (w67:T12)
            n331 = control-ref of="Modules Tree"() -> (w66:refnum<vi>)
            n332 = call "Set Tree custom symbols.vi"("TreeControl in"=w66) -> ("TreeControl out"=w65:refnum<vi>)  [unwired: 10 in]
          }
          event User Event {
            n333 = event-data() -> ("Projects"=w76:string[])  [unwired: 1 in]
            n334 = Array Size(array=w76) -> (size(s)=w75:i32)
            n335 = Equal?(x=1, y=w75) -> (x = y?=w73:bool)
            n336 = control-ref of="Projects"() -> (w77:refnum<vi>)
            n337 = case shown="False" w73 {
              tunnel: w77 -> [w83 w86]
              tunnel: w76 -> [w82 w85]
              frame True {
                n338 = Index Array(array=w82) -> (element=w81:string)  [unwired: 1 in]
                n339 = property class="CmbBox"(reference=w83, "Strings[]"=w82, "Val(Sgnl)"=w81) -> ()  [unwired: 1 in, 2 out]
              }
              frame False {
                n340 = property class="CmbBox"(reference=w86, "Strings[]"=w85, "Text.Text"="") -> ()  [unwired: 1 in, 2 out]
              }
            }
          }
          event User Event {
            n341 = event-data() -> ("Targets"=w88:string[])  [unwired: 1 in]
            n342 = Index Array(array=w88) -> (element=w87:string)  [unwired: 1 in]
            n343 = control-ref of="Targets"() -> (w90:refnum<vi>)
            n344 = property class="CmbBox"(reference=w90, "Strings[]"=w88, "Value"=w87) -> ()  [unwired: 1 in, 2 out]
          }
          event User Event {
            n345 = event-data() -> ("Progress"=→"Progress":u16)  [unwired: 1 in]
          }
          event Mouse Enter {
            n346 = event-data() -> ("CtlRef"=w97:refnum<vi>)  [unwired: 1 in]
            n347 = property class="Ctl"(reference=w97) -> ("Label.Text"=w103:string, "TipStrip"=w104:string)  [unwired: 1 in, 2 out]
            n348 = control-ref of="antidoc"() -> (w98:refnum<vi>)
            n349 = control-ref of="Panther Indicator"() -> (w102:refnum<vi>)
            n350 = control-ref of="Process Indicator"() -> (w101:refnum<vi>)
            n351 = control-ref of="Event Indicator"() -> (w100:refnum<vi>)
            n352 = Empty String/Path?(string/path=w104) -> (empty?=w105:bool)
            n353 = Build Array(w98, w102, w101, w100) -> (w99:refnum<vi>[])
            n354 = call "Set Indicators Visibility Status.vi"("Indicator Refs"=w99, "Label"=w103) -> ()  [unwired: 10 in]
            n355 = case shown="False" w105 {
              tunnel: w104 -> [w109 _]
              frame False {
                n356 = call "Status Updated.vi"("Status"=w109) -> ()  [unwired: 10 in, 1 out]
              }
              frame True {
              }
            }
          }
          event User Event {
            n357 = event-data() -> ()  [unwired: 1 in, 1 out]
            n358 = control-ref of="This VI"() -> (w111:refnum<vi>)
            n359 = property class="VI"(reference=w111) -> ("Panel"=w112:refnum<vi>)  [unwired: 1 in, 2 out]
            n360 = property class="Pnl"(reference=w112) -> ("Controls[]"=w110:refnum<vi>[])  [unwired: 1 in, 2 out]
            n361 = register-events(reference=w115, w110) -> (reference out=w113:refnum<event-registration>)  [unwired: 3 in, 1 out]
          }
          event User Event {
            n362 = event-data() -> ("Scale Max"=w119:i32)  [unwired: 1 in]
            n363 = control-ref of="Progress"() -> (w118:refnum<vi>)
            n364 = property class="Slide (strict)"(reference=w118, "Scale.Maximum"=w119) -> (error out=w123:errorcluster)  [unwired: 1 in, 1 out]
          }
          event User Event {
            n365 = event-data() -> ("Module Type"=w130:T10)  [unwired: 1 in]
            n366 = Equal?(x=Module_type--enum."Module type: Cloneable", y=w130) -> (x = y?=w128:bool)
            n367 = Select(t=T13."Enabled" ("Disabled"), s=w128, f=T13."Disabled and Grayed Out") -> (s? t:f=w125:T13)
            n368 = control-ref of="Module ID"() -> (w127:refnum<vi>)
            n369 = property class="DigNum (strict)"(reference=w127, "DisabledEnum"=w125) -> ()  [unwired: 1 in, 2 out]
          }
          event User Event {
            n370 = event-data() -> ("Status"=→"Status":string)  [unwired: 1 in]
          }
        }
        n371 = call-dynamic "Delacor_lib_QMH_Error Handler - Helper Loop.vi"("error in"=w54, "Message Queue in"=w45) -> ("dup error in"=w53:errorcluster)  [unwired: 8 in, 1 out]
      }
    }
    frame Error {
      # "Synchronize Caller Events.vi will inform Start Module.vi that the module has launched and will let the code calling Start Module.vi register for broadcasts and would permit the caller receive the broadcast that an error occurred at launch time."
      n372 = call-dynamic "Delacor_lib_QMH_Release Message Queue.vi"("error in"=w852, "Message Queue"=w846) -> ("error out"=w851:errorcluster)  [unwired: 9 in]
      n373 = call "Synchronize Caller Events.vi"("Singleton Module Admin in"=w847) -> ("error out"=w853:errorcluster)  [unwired: 9 in, 1 out]
      n374 = call "Module Name--constant.vi"() -> ("Module Name"=w849:string)  [unwired: 11 in]
      n375 = Format Into String(format string="An error occurred during initialization. %s is no longer running.", w849) -> (resulting string=w844:string)  [unwired: 2 in, 1 out]
      n376 = Merge Errors(w851, w853) -> (w854:errorcluster)
      n377 = call "Stop Module.vi"("Origin"=w844) -> ()  [unwired: 10 in, 1 out]
      n378 = call "Error Reported.vi"("Additional Information"=w844, "Error"=w854) -> ()  [unwired: 9 in, 1 out]
    }
  }
  n379 = Merge Errors(w26, w28, w21) -> (w25:errorcluster)
  n380 = call "Close Module.vi"("error in (no error)"=w25, "Module Admin in"=w16) -> ("error out"=w27:errorcluster, "External Launch"=w10:bool, "Module Admin out"=w11:refnum<class "Delacor_lib_QMH_Module Admin.lvclass">)  [unwired: 7 in]
  n381 = Unregister For Events(event registration refnum=w8) -> ()  [unwired: 1 in, 1 out]
  n382 = Unregister For Events(event registration refnum=w15, error in=w27) -> (error out=w24:errorcluster)
  "error out" <- w24
  n383 = case "External Launch?" shown="True" w10 {
    tunnel: w24 -> [_ w855]
    frame False {
    }
    frame True {
      n384 = case shown="No Error" w855 {
        frame No Error {
          n385 = invoke class="VI" method="FP.Close"() -> ()  [unwired: 3 in, 3 out]
        }
        frame Error {
          n386 = invoke on="Invoke Node" class="VI" method="FP.Open"("Activate"=TRUE ("Activate?")) -> ()  [unwired: 4 in, 5 out]
        }
      }
    }
  }
  n387 = local write "Module Admin"(w11) -> ()
  n388 = call "Update Window Position.vi"("Window Position"=Window_Position--enum."Right") -> ()  [unwired: 10 in, 1 out]
  n389 = call "Status Updated.vi"("Status"="pues si me iniciaton") -> ()  [unwired: 10 in, 1 out]
